vi "vacuum.vi"() -> ()   [LabVIEW 2014, in "Panels.lvlib"]
uses:
  Panels.lvlib
  CSlibraries-extern/DimLVEvent/DimIndicators/DimIndicators.lvlib
  CSCore/CSSystem/CoreLib/CoreLib.lvlib
  CSlibraries/UtilityLib/UtilityLib.valueStatus.ctl
  CSlibraries/UtilityLib/UtilityLib.lvlib
  CSCore/CSSystem/CoreLib/CoreLib.short 2 byte array.vi
  Instance           1 14Saved   vacuum .vi
  Instance           2 14Saved   vacuum .vi
  Instance           3 14Saved   vacuum .vi
  Instance           4 14Saved   vacuum .vi
  Instance           5 14Saved   vacuum .vi
  CSlibraries-extern/DimLVEvent/LVDimInterface/LVDimInterface.lvlib
  CSCore/CSSystem/CoreLib/CoreLib.string 2 byte array.vi
  CSCore/BaseProcess/BaseProcess.descriptor string definition.ctl
  CSCore/BaseProcess/BaseProcess.lvlib
  CSCore/CSSystem/CoreDefs/CoreDefs.rawDataType.ctl
  CSCore/CSSystem/CoreDefs/CoreDefs.call_type.ctl
  CSlibraries-extern/DimLVEvent/DimIndicators/DimIndicators.numericType.ctl
  CSlibraries-extern/DimLVEvent/DimIndicators/DimIndicators.numericArrayType.ctl
  CSlibraries-extern/DimLVEvent/DimIndicators/DimIndicators.anyType.ctl
panel:
  out "i ref out":refnum<vi>
  out "i ref out":refnum<vi>
  out "BOB1TP":bool
  out "BOB1TPen":bool
  in  "BOB2TISout_MonData":T1
  in  "BOB2TISin_MonData":T1
  out "BOB2TIS":bool
  in  "FVCPIR_MonData":T1={"data"=inf, "no link"=FALSE, "quality"=1, "timeStamp"=3265900746.554}
  out "FVCPIR":dbl=inf format="%.2e"
  out "LHeLevel":dbl=inf format="%.4f"
  out "LN2Level":dbl=inf format="%.4f"
  in  "LN2Level_MonData":T1={"data"=inf, "no link"=FALSE, "quality"=1, "timeStamp"=3265900746.538}
  in  "LHeLevel_MonData":T1={"data"=inf, "no link"=FALSE, "quality"=1, "timeStamp"=3265900746.554}
  in  "call cluster in":T2={"Object"="", "Selector"="", "CallType"=enum."synchronous", "Async Object"="", "Async Selector"="", "Data Descriptor"="", "Data"=[], "Error #"=0, "Expire"=0}
  in  "ReasonForLocking_SetData":T5
  in  "call cluster in":T2={"Object"="", "Selector"="", "CallType"=enum."synchronous", "Async Object"="", "Async Selector"="", "Data Descriptor"="", "Data"=[], "Error #"=0, "Expire"=0}
  in  "Reason for locking":string
  in  "BOB6_MCP_SetData":T6={"data"=[0.0, 0.0, 0.0, 0.0], "no link"=FALSE, "quality"=1, "timeStamp"=3270208307.575}
  in  "BOB6_Pho_SetData":T6={"data"=[0.0, 0.0, 0.0, 0.0], "no link"=FALSE, "quality"=1, "timeStamp"=3270208307.575}
  in  "BOB5_MCP_SetData":T6={"data"=[0.0, 0.0, 0.0, 0.0], "no link"=FALSE, "quality"=1, "timeStamp"=3270208307.575}
  in  "BOB5_Pho_SetData":T6={"data"=[0.0, 0.0, 0.0, 0.0], "no link"=FALSE, "quality"=1, "timeStamp"=3270208307.575}
  in  "BOB3_MCP_SetData":T6={"data"=[0.0, 0.0, 0.0, 0.0], "no link"=FALSE, "quality"=1, "timeStamp"=3270208307.575}
  in  "BOB3_Pho_SetData":T6={"data"=[0.0, 0.0, 0.0, 0.0], "no link"=FALSE, "quality"=1, "timeStamp"=3270208307.591}
  in  "N4VAC_MonData":T1
  in  "CB5SAFE_MonData":T1
  in  "FVAPIR_MonData":T1={"data"=inf, "no link"=FALSE, "quality"=1, "timeStamp"=3265900746.538}
  in  "FVBPIR_MonData":T1={"data"=inf, "no link"=FALSE, "quality"=1, "timeStamp"=3265900746.554}
  in  "BOB6_Pho_MonData":T1={"data"=inf, "no link"=FALSE, "quality"=1, "timeStamp"=3265900746.538}
  in  "BOB5PIR_MonData":T1={"data"=inf, "no link"=FALSE, "quality"=1, "timeStamp"=3265900746.538}
  in  "PT1PEN_MonData":T1={"data"=inf, "no link"=FALSE, "quality"=1, "timeStamp"=3265900746.538}
  in  "PT1PIR_MonData":T1={"data"=inf, "no link"=FALSE, "quality"=1, "timeStamp"=3265900746.522}
  in  "BOB6_MCP_MonData":T1={"data"=inf, "no link"=FALSE, "quality"=1, "timeStamp"=3265900746.554}
  in  "PT2PIR_MonData":T1={"data"=inf, "no link"=FALSE, "quality"=1, "timeStamp"=3265900746.569}
  in  "PT2PEN_MonData":T1={"data"=inf, "no link"=FALSE, "quality"=1, "timeStamp"=3265900746.554}
  in  "BOB1PEN_MonData":T1={"data"=inf, "no link"=FALSE, "quality"=1, "timeStamp"=3265900746.538}
  in  "BOB1PIR_MonData":T1={"data"=inf, "no link"=FALSE, "quality"=1, "timeStamp"=3265900746.569}
  in  "BOB2PEN_MonData":T1={"data"=inf, "no link"=FALSE, "quality"=1, "timeStamp"=3265900746.554}
  in  "BOB2PIR_MonData":T1={"data"=inf, "no link"=FALSE, "quality"=1, "timeStamp"=3265900746.538}
  in  "BOB3PEN_MonData":T1={"data"=inf, "no link"=FALSE, "quality"=1, "timeStamp"=3265900746.569}
  in  "BOB5PEN_MonData":T1={"data"=inf, "no link"=FALSE, "quality"=1, "timeStamp"=3265900746.569}
  in  "BOB5_Pho_MonData":T1={"data"=inf, "no link"=FALSE, "quality"=1, "timeStamp"=3265900746.538}
  in  "BOB5_MCP_MonData":T1={"data"=inf, "no link"=FALSE, "quality"=1, "timeStamp"=3265900746.585}
  in  "BOB4PIR_MonData":T1={"data"=inf, "no link"=FALSE, "quality"=1, "timeStamp"=3265900746.538}
  in  "BOB4PEN_MonData":T1={"data"=inf, "no link"=FALSE, "quality"=1, "timeStamp"=3265900746.554}
  in  "CB3PEN_MonData":T1={"data"=inf, "no link"=FALSE, "quality"=1, "timeStamp"=3265900746.569}
  in  "CB2PEN_MonData":T1={"data"=inf, "no link"=FALSE, "quality"=1, "timeStamp"=3265900746.522}
  in  "CB1PEN_MonData":T1={"data"=inf, "no link"=FALSE, "quality"=1, "timeStamp"=3265900746.538}
  in  "BOB3_Pho_MonData":T1={"data"=inf, "no link"=FALSE, "quality"=1, "timeStamp"=3265900746.6}
  in  "BOB3_MCP_MonData":T1={"data"=inf, "no link"=FALSE, "quality"=1, "timeStamp"=3265900746.585}
  in  "BOB3PIR_MonData":T1={"data"=inf, "no link"=FALSE, "quality"=1, "timeStamp"=3265900746.569}
  out "FVAPIR":dbl=inf format="%.2e"
  out "FVBPIR":dbl=inf format="%.2e"
  out "BOB6_Pho":dbl=inf format="%.3f"
  out "BOB6_MCP":dbl=inf format="%.3f"
  out "PT1PIR":dbl=inf format="%.2e"
  out "PT1PEN":dbl=inf format="%.2e"
  out "PT2PIR":dbl=inf format="%.2e"
  out "PT2PEN":dbl=inf format="%.2e"
  out "BOB5_Pho":dbl=inf format="%.3f"
  out "BOB5_MCP":dbl=inf format="%.3f"
  out "BOB5PIR":dbl=inf format="%.2e"
  out "BOB5PEN":dbl=inf format="%.2e"
  out "BOB4PIR":dbl=inf format="%.2e"
  out "BOB4PEN":dbl=inf format="%.2e"
  out "CB3PEN":dbl=inf format="%.2e"
  out "CB2PEN":dbl=inf format="%.2e"
  out "CB1PEN":dbl=inf format="%.2e"
  out "BOB3_Pho":dbl=inf format="%.3f"
  out "BOB3_MCP":dbl=inf format="%.3f"
  out "BOB3PIR":dbl=inf format="%.2e"
  out "BOB3PEN":dbl=inf format="%.2e"
  out "BOB2PIR":dbl=inf format="%.2e"
  out "BOB2PEN":dbl=inf format="%.2e"
  out "BOB1PIR":dbl=inf format="%.2e"
  out "BOB1PEN":dbl=inf format="%.2e"
  in  "BOB1FVAout_MonData":T1
  in  "BOB1FVBout_MonData":T1
  in  "BOB1GVPout_MonData":T1
  in  "BOB1GVSout_MonData":T1
  in  "BOB1BETAout_MonData":T1
  in  "BOB1TPout_MonData":T1
  in  "BOB2FCout_MonData":T1
  in  "BOB2FVAout_MonData":T1
  in  "BOB1FCout_MonData":T1
  in  "BOB2FVBout_MonData":T1
  in  "BOB2GVPout_MonData":T1
  in  "BOB2GVSout_MonData":T1
  in  "BOB2TPout_MonData":T1
  in  "TSTGVSout_MonData":T1
  in  "TSTTPout_MonData":T1
  in  "TSTFVAout_MonData":T1
  in  "TSTFVBout_MonData":T1
  in  "BOB3GVSout_MonData":T1
  in  "BOB3GVPout_MonData":T1
  in  "BOB3TPout_MonData":T1
  in  "BOB3FCout_MonData":T1
  in  "BOB3MCPout_MonData":T1
  in  "BOB3FVAout_MonData":T1
  in  "BOB3FVBout_MonData":T1
  in  "CBFVAout_MonData":T1
  in  "CBFVBout_MonData":T1
  in  "CBFVCout_MonData":T1
  in  "CB1TPout_MonData":T1
  in  "CB2TPout_MonData":T1
  in  "CB3TPout_MonData":T1
  in  "CB4TPout_MonData":T1
  in  "CB5GVSout_MonData":T1
  in  "BOB4GVSout_MonData":T1
  in  "BOB4GVPout_MonData":T1
  in  "BOB4TPout_MonData":T1
  in  "BOB4BETAout_MonData":T1
  in  "BOB4FVAout_MonData":T1
  in  "BOB4FVBout_MonData":T1
  in  "BOB5GVSout_MonData":T1
  in  "BOB5GVPout_MonData":T1
  in  "BOB5TPout_MonData":T1
  in  "BOB5FCout_MonData":T1
  in  "BOB5MCPout_MonData":T1
  in  "BOB5FVAout_MonData":T1
  in  "BOB5FVBout_MonData":T1
  in  "PT1GVPout_MonData":T1
  in  "PT1TPout_MonData":T1
  in  "PT1FVAout_MonData":T1
  in  "PT1FVBout_MonData":T1
  in  "PT2GVPout_MonData":T1
  in  "PT2TPout_MonData":T1
  in  "PT2FVAout_MonData":T1
  in  "PT2FVBout_MonData":T1
  in  "BOB2lock_SetData":T1
  in  "BOB3lock_SetData":T1
  in  "BOB4lock_SetData":T1
  in  "BOB5lock_SetData":T1
  in  "TSTlock_SetData":T1
  in  "CBlock_SetData":T1
  in  "PTlock_SetData":T1
  in  "BOB1lock_SetData":T1
  in  "PT2FVBin_MonData":T1
  in  "PT2FVAin_MonData":T1
  in  "PT2TPin_MonData":T1
  in  "PT2GVPin_MonData":T1
  in  "PT1FVBin_MonData":T1
  in  "PT1FVAin_MonData":T1
  in  "PT1TPin_MonData":T1
  in  "PT1GVPin_MonData":T1
  in  "BOB5FVBin_MonData":T1
  in  "BOB5FVAin_MonData":T1
  in  "BOB5MCPin_MonData":T1
  in  "BOB5FCin_MonData":T1
  in  "BOB5TPin_MonData":T1
  in  "BOB5GVPin_MonData":T1
  in  "BOB5GVSin_MonData":T1
  in  "BOB4FVBin_MonData":T1
  in  "BOB4FVAin_MonData":T1
  in  "BOB4BETAin_MonData":T1
  in  "BOB4TPin_MonData":T1
  in  "BOB4GVPin_MonData":T1
  in  "BOB4GVSin_MonData":T1
  in  "CB5GVSin_MonData":T1
  in  "CB4TPin_MonData":T1
  in  "CB3TPin_MonData":T1
  in  "CB2TPin_MonData":T1
  in  "CB1TPin_MonData":T1
  in  "CBFVCin_MonData":T1
  in  "CBFVBin_MonData":T1
  in  "CBFVAin_MonData":T1
  in  "BOB3FVBin_MonData":T1
  in  "BOB3FVAin_MonData":T1
  in  "BOB3MCPin_MonData":T1
  in  "BOB3FCin_MonData":T1
  in  "BOB3TPin_MonData":T1
  in  "BOB3GVPin_MonData":T1
  in  "BOB3GVSin_MonData":T1
  in  "TSTFVBin_MonData":T1
  in  "TSTFVAin_MonData":T1
  in  "TSTTPin_MonData":T1
  in  "TSTGVSin_MonData":T1
  in  "BOB2TPin_MonData":T1
  out "TSTlock":bool
  out "BOB3lock":bool
  out "BOB1BETA":bool
  out "BOB1FC":bool
  out "BOB6FC":bool
  out "BOB6MCP":bool=TRUE
  out "BOB3MCP":bool
  out "BOB3FC":bool
  out "BOB2FC":bool
  out "BOB1lock":bool
  out "BOB2lock":bool
  out "BOB5MCP":bool
  out "BOB5FC":bool
  out "BOB4BETA":bool
  out "CBlock":bool
  out "PTlock":bool
  out "BOB5lock":bool
  out "BOB4lock":bool
  out "BOB1GVS":bool
  out "TSTGVS":bool
  out "BOB2GVS":bool
  out "BOB3GVS":bool
  out "BOB4GVS":bool
  out "BOB5GVS":bool
  out "BOB1GVP":bool
  out "BOB2GVP":bool
  out "BOB3GVP":bool
  out "CB5GVS":bool
  out "BOB4GVP":bool
  out "BOB5GVP":bool
  out "PT1GVP":bool
  out "PT2GVP":bool
  out "BOB1FVA":bool
  out "BOB1FVB":bool
  out "BOB2FVA":bool
  out "BOB2FVB":bool
  out "TSTFVA":bool
  out "TSTFVB":bool
  out "BOB3FVA":bool
  out "BOB3FVB":bool
  out "CBFVA":bool
  out "CBFVC":bool
  out "CBFVB":bool
  out "BOB4FVA":bool
  out "BOB4FVB":bool
  out "BOB5FVA":bool
  out "BOB5FVB":bool
  out "PT1FVA":bool
  out "PT1FVB":bool
  out "PT2FVA":bool
  out "PT2FVB":bool
  out "CB1TP":bool
  out "BOB3TP":bool
  out "TSTTP":bool
  out "CB2TP":bool
  out "BOB2TP":bool
  out "CB5SAFE":bool=TRUE
  out "N4VAC":bool=TRUE
  out "BOB5TP":bool
  out "PT2TP":bool
  out "BOB4TP":bool
  out "PT1TP":bool
  out "CB4TP":bool
  out "CB3TP":bool
  in  "BOB2GVSin_MonData":T1
  in  "BOB2GVPin_MonData":T1
  out "i ref out":refnum<vi>
  in  "BOB1FCin_MonData":T1
  in  "BOB2FVAin_MonData":T1
  in  "BOB2FCin_MonData":T1
  in  "BOB1TPin_MonData":T1
  in  "BOB1BETAin_MonData":T1
  in  "BOB1GVSin_MonData":T1
  in  "BOB1GVPin_MonData":T1
  in  "BOB1FVBin_MonData":T1
  in  "BOB1FVAin_MonData":T1
  in  "BOB2FVBin_MonData":T1
  out "PT2FVBen":bool
  out "PT2FVAen":bool
  out "PT1FVBen":bool
  out "PT1FVAen":bool
  out "BOB5FVBen":bool
  out "BOB5FVAen":bool
  out "BOB4FVBen":bool
  out "BOB4FVAen":bool
  out "BOB3FVBen":bool
  out "BOB3FVAen":bool
  out "TSTFVBen":bool
  out "BOB2FVBen":bool
  out "TSTFVAen":bool
  out "BOB2FVAen":bool
  out "BOB1FVBen":bool
  out "BOB1FVAen":bool
  out "CBFVCen":bool
  out "CBFVBen":bool
  out "CBFVAen":bool
  out "PT2GVPen":bool
  out "PT1GVPen":bool
  out "BOB5GVPen":bool
  out "BOB4GVPen":bool
  out "BOB3GVPen":bool
  out "BOB2GVPen":bool
  out "BOB1GVPen":bool
  out "BOB5GVSen":bool
  out "BOB4GVSen":bool
  out "BOB3GVSen":bool
  out "BOB2GVSen":bool
  out "BOB1GVSen":bool
  out "TSTGVSen":bool
  out "BOB2TPen":bool
  out "TSTTPen":bool
  out "BOB3TPen":bool
  out "BOB4TPen":bool
  out "BOB5TPen":bool
  out "PT1TPen":bool
  out "PT2TPen":bool
  out "CB1TPen":bool
  out "CB5GVSen":bool
  # "voltage"
  # "V"
  # "voltage"
  # "V"
  # "N4VAC"
  # "CB5SAFE"
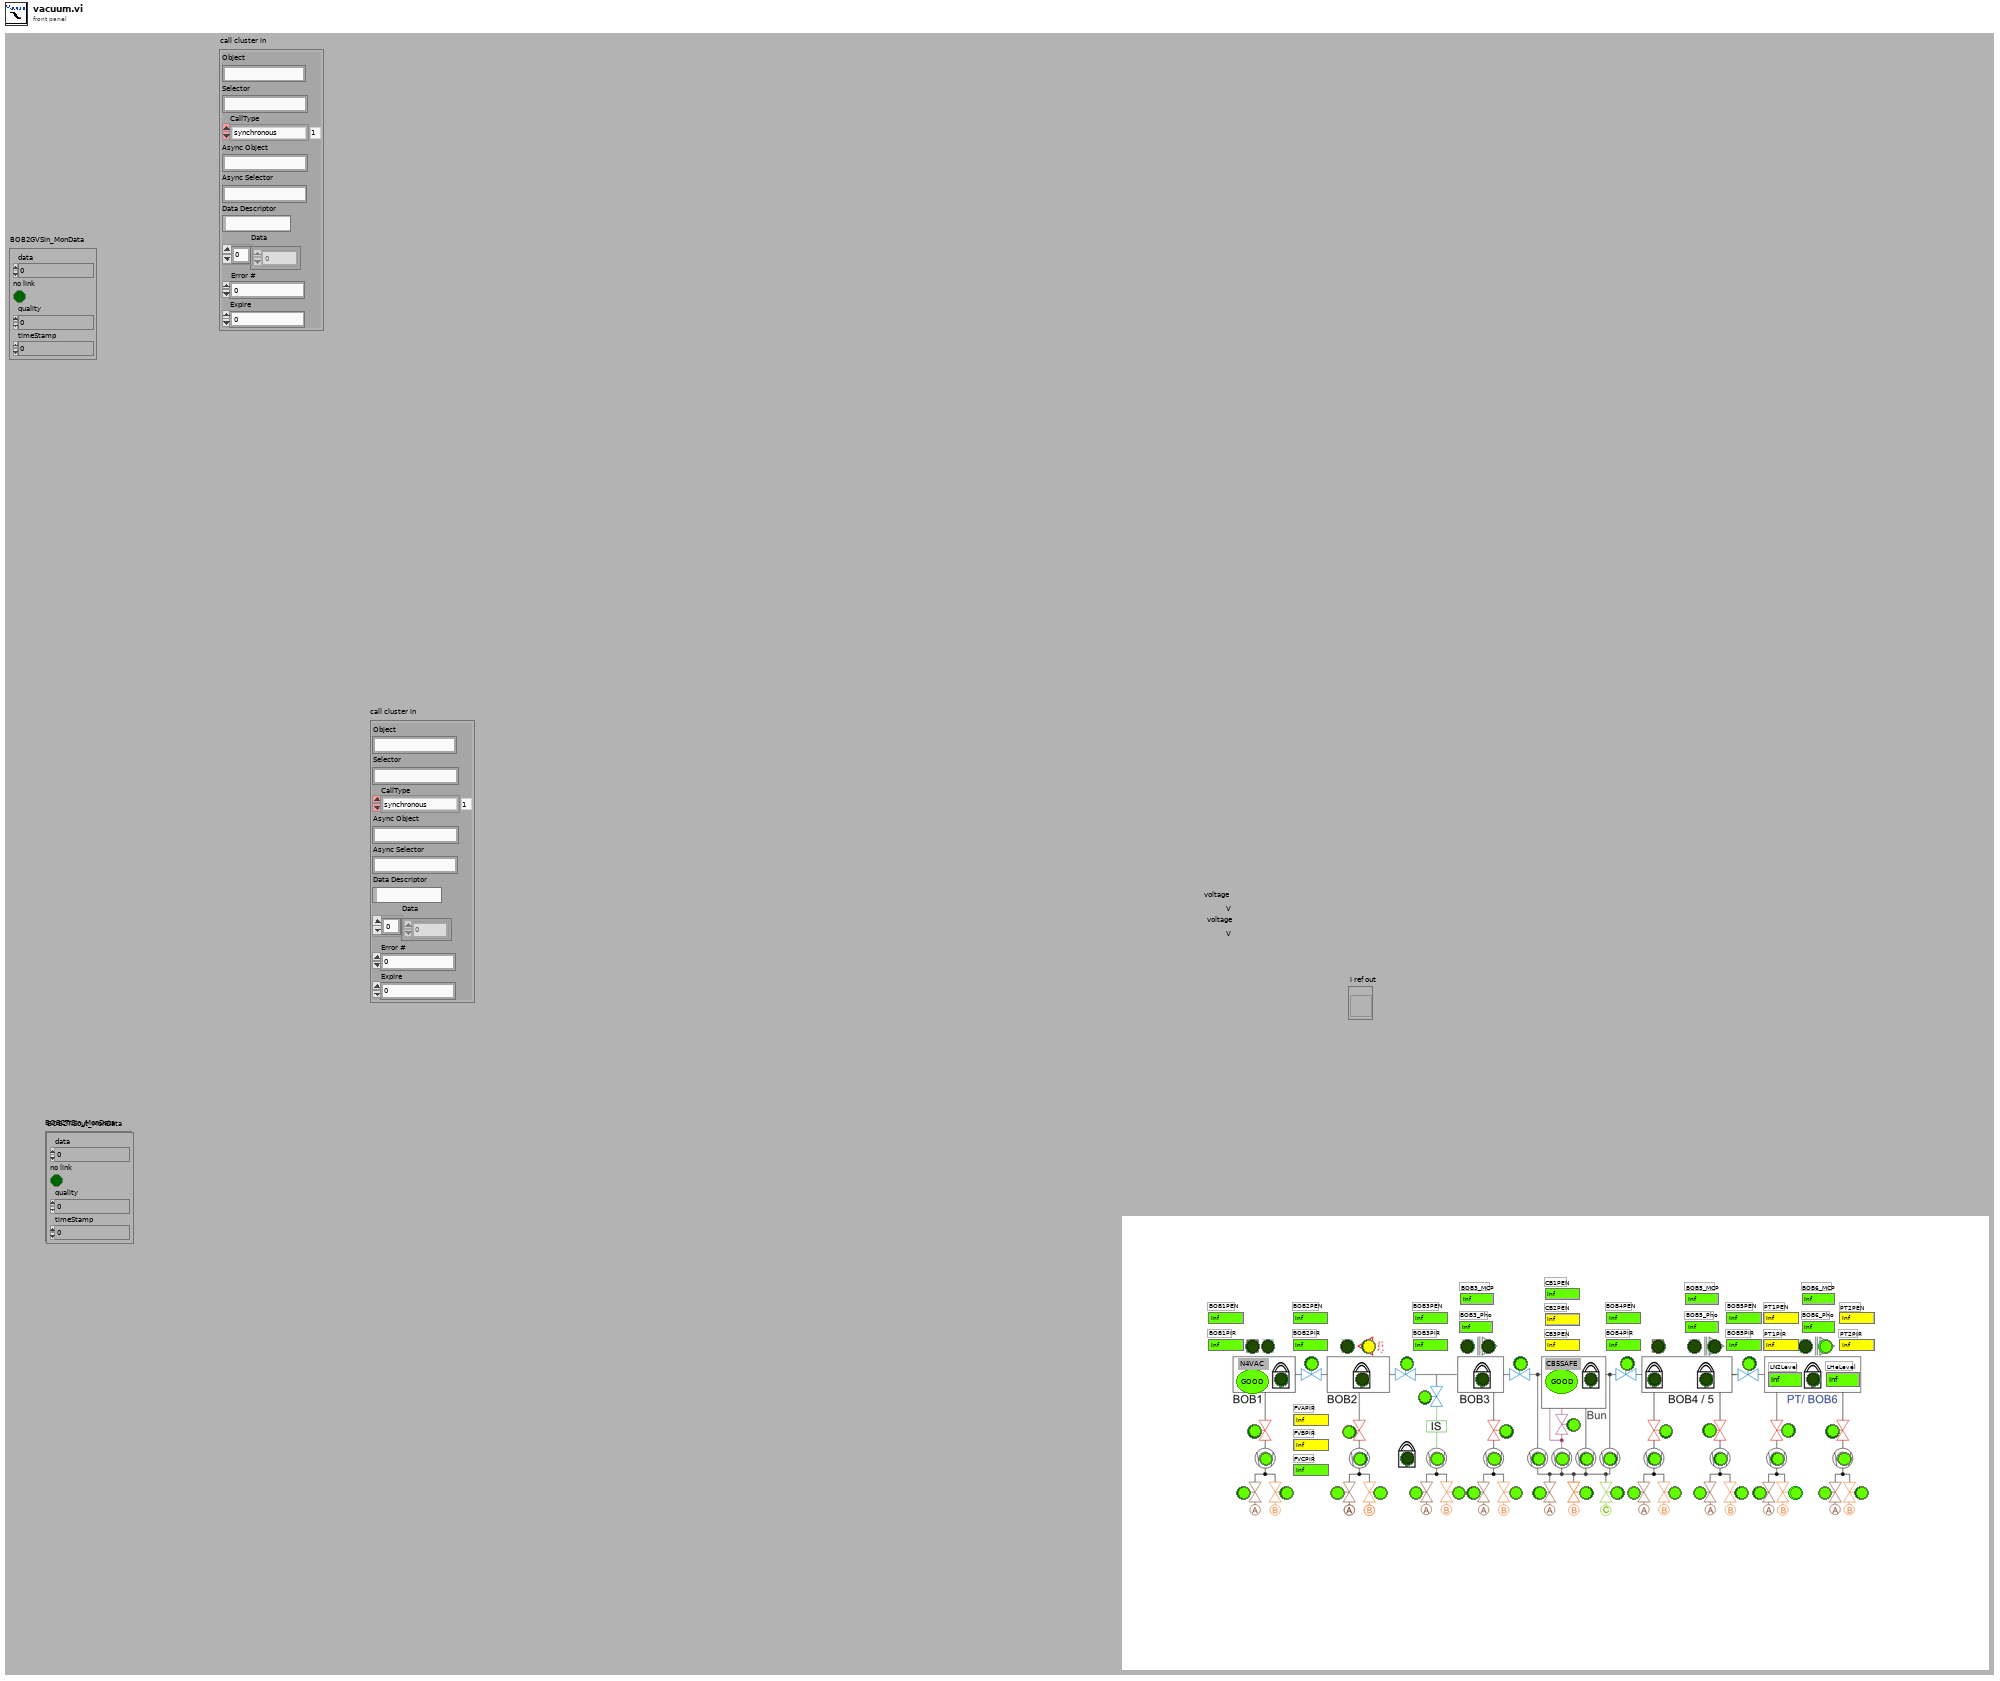
[diagram p1: front panel]
types:
  T1 = typedef "DimIndicators.lvlib/DimIndicators.numericType.ctl" = cluster{"data":dbl, "no link":bool, "quality":i32, "timeStamp":dbl}
  T2 = typedef "CoreDefs.call_type.ctl" = cluster{"Object":string, "Selector":string, "CallType":enum16{"simple", "synchronous", "asynchronous"}, "Async Object":string, "Async Selector":string, "Data Descriptor":T3, "Data":T4, "Error #":i32, "Expire":u32}
  T3 = typedef "BaseProcess.lvlib/BaseProcess.descriptor string definition.ctl" = string
  T4 = typedef "CoreDefs.rawDataType.ctl" = i8[]
  T5 = typedef "DimIndicators.lvlib/DimIndicators.anyType.ctl" = cluster{"data":string, "no link":bool, "quality":i32, "timeStamp":dbl}
  T6 = typedef "DimIndicators.lvlib/DimIndicators.numericArrayType.ctl" = cluster{"data":dbl[], "no link":bool, "quality":i32, "timeStamp":dbl}
  T7 = typedef "UtilityLib.lvlib/UtilityLib.valueStatus.ctl" = enum16{"no info available", "stand by/off", "on", "warning", "alarm/malfunction", "not implemented", "user action required", "important information", "system default", "control default", "indicator default", "button default"}
  T8 = cluster{"data":i16, "no link":bool, "quality":i32, "timeStamp":dbl}
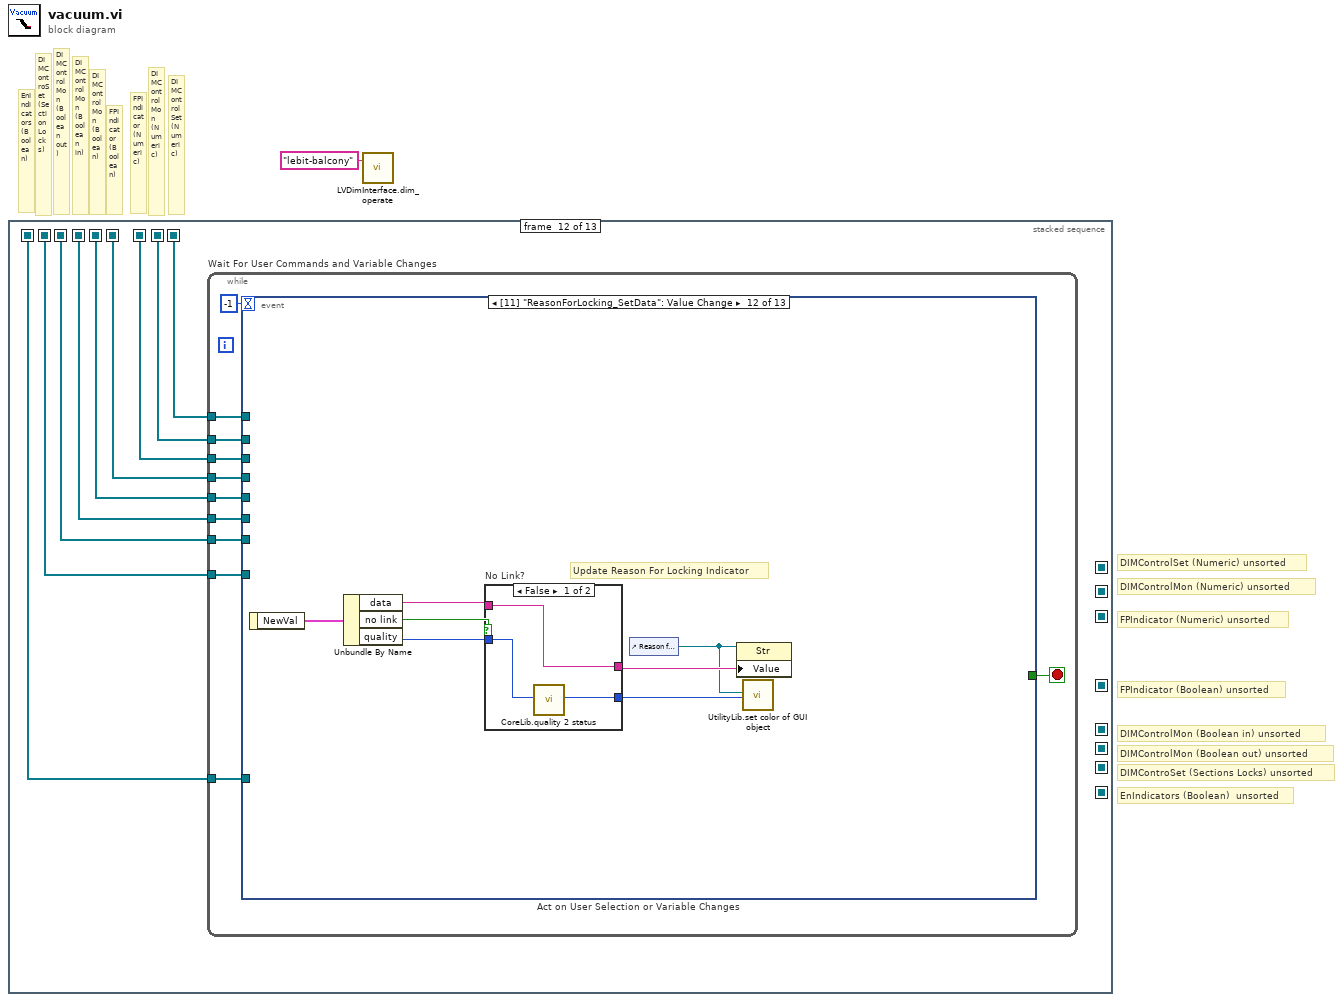
[diagram p0: block diagram]
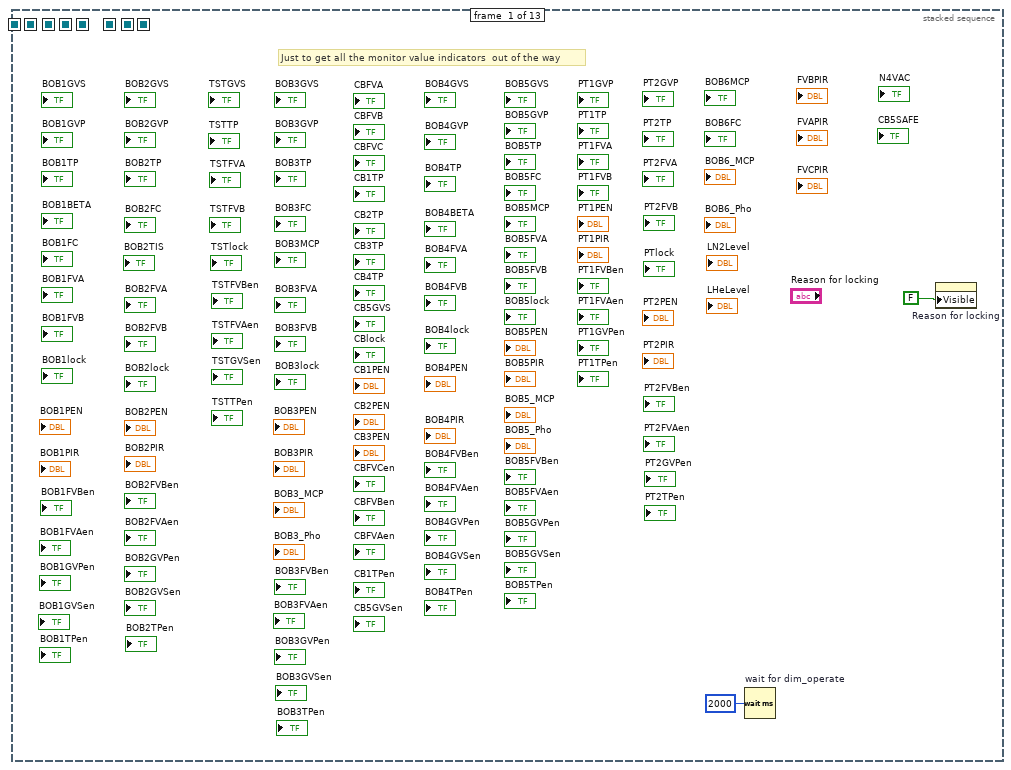
[diagram p2: hidden frame]
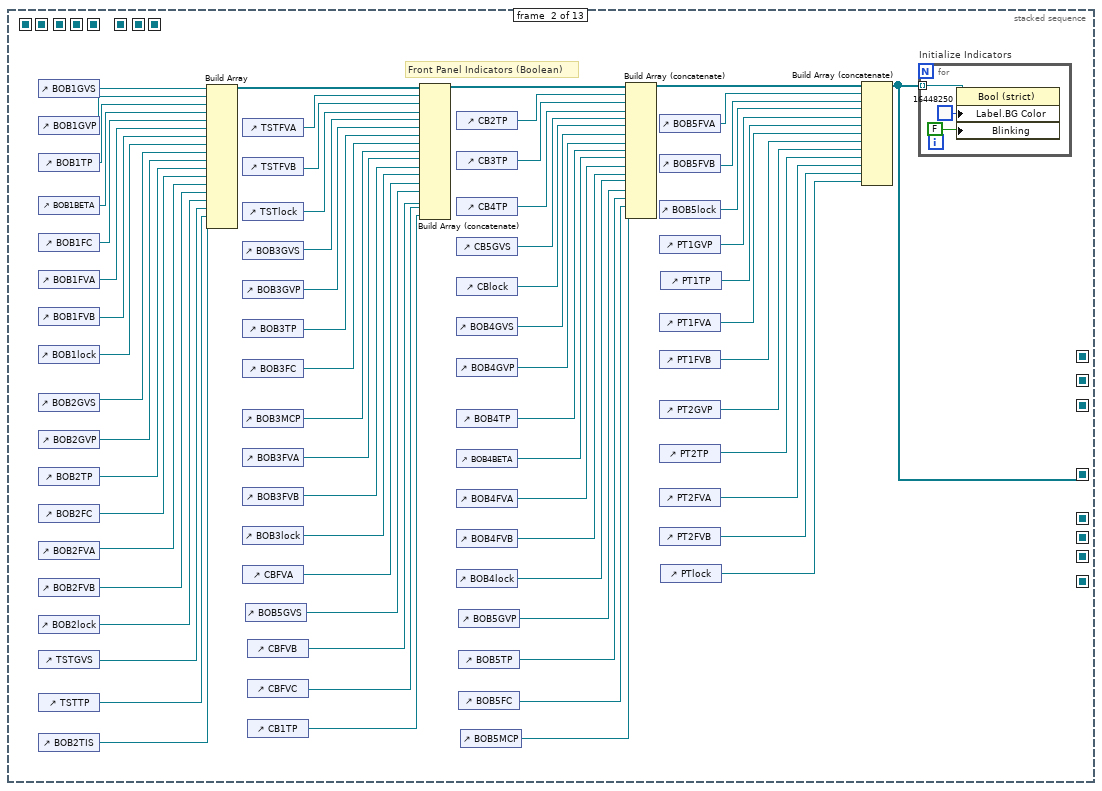
[diagram p3: hidden frame]
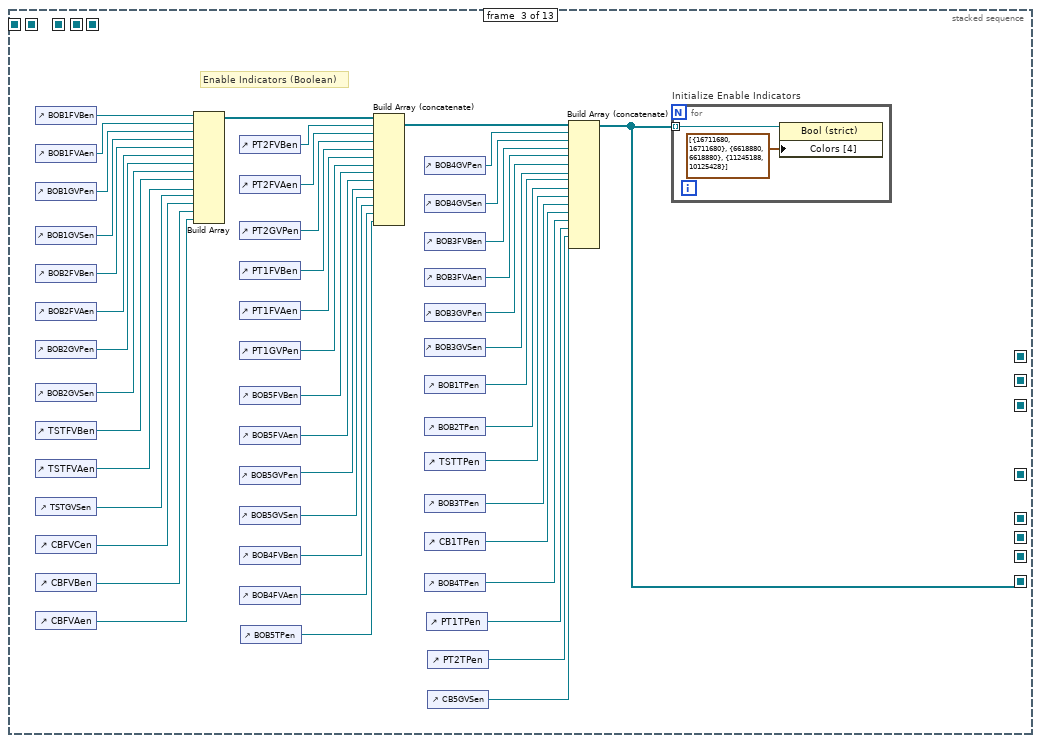
[diagram p4: hidden frame]
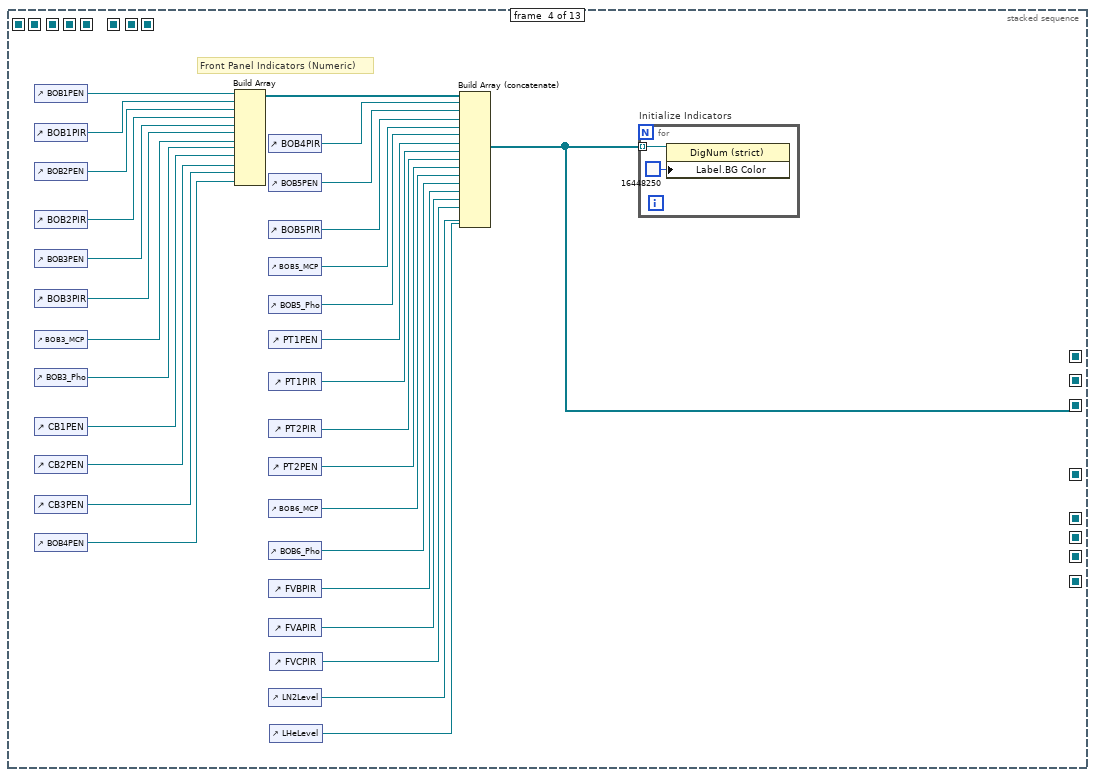
[diagram p5: hidden frame]
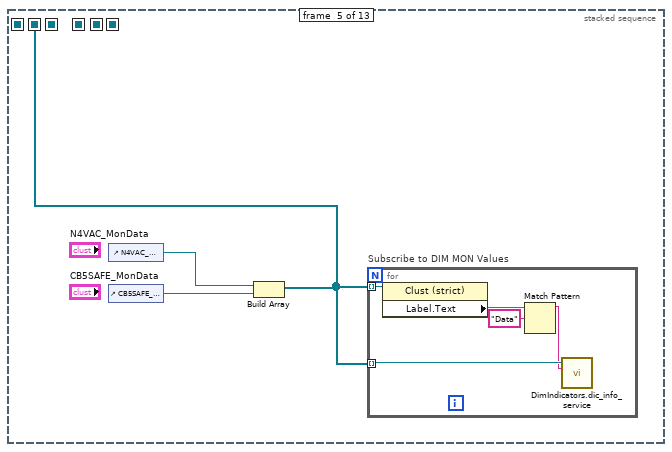
[diagram p6: hidden frame]
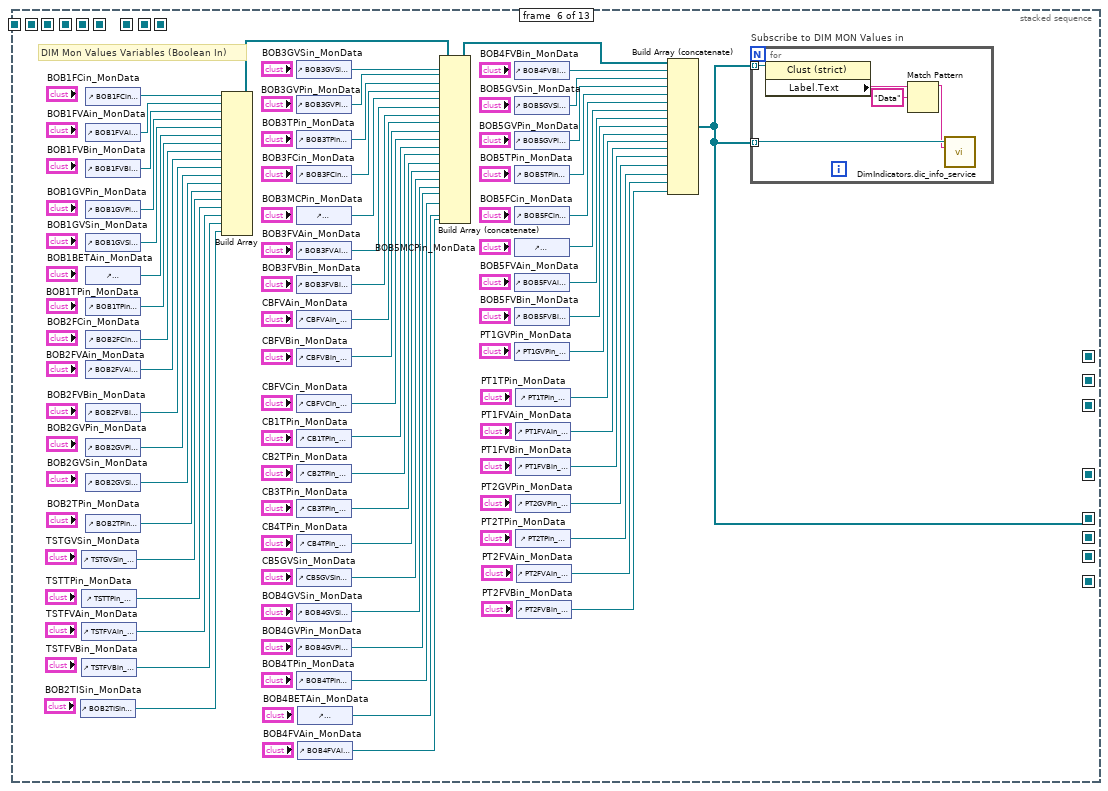
[diagram p7: hidden frame]
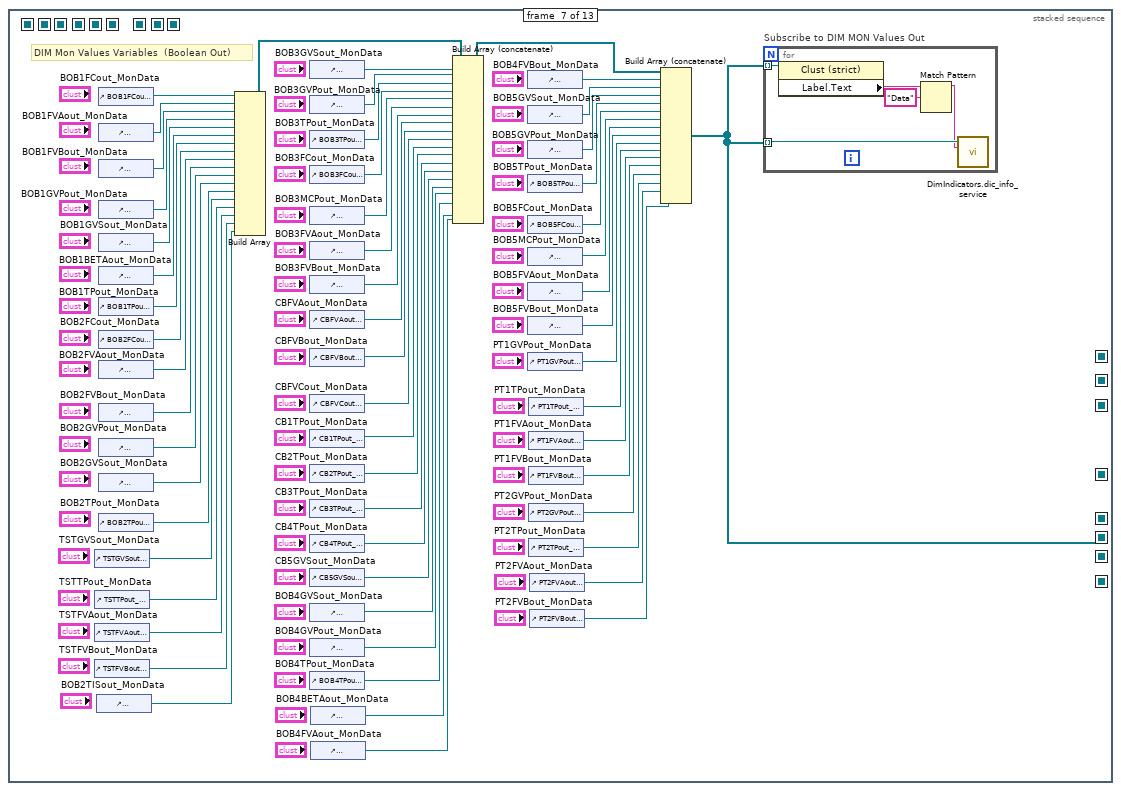
[diagram p8: hidden frame]
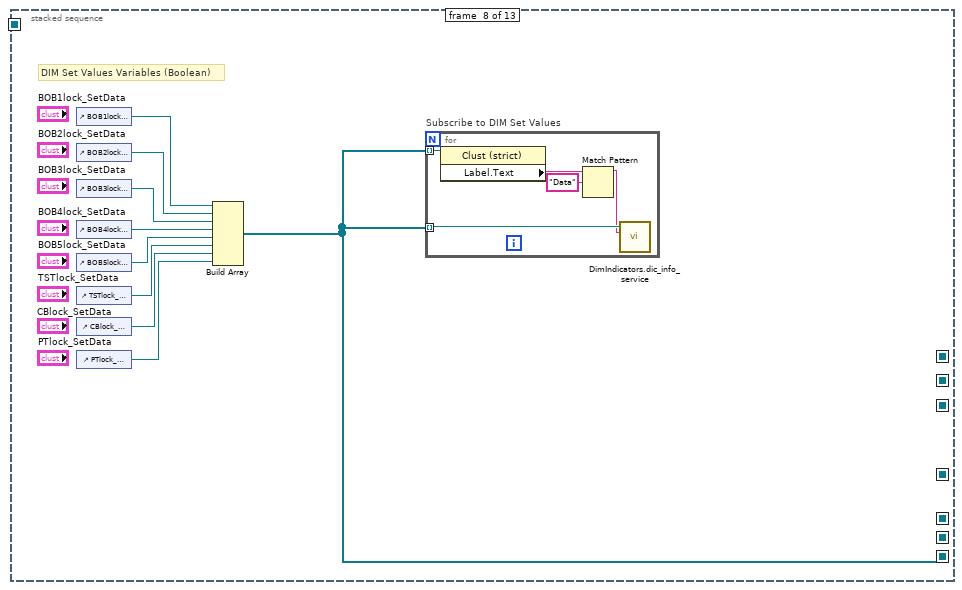
[diagram p9: hidden frame]
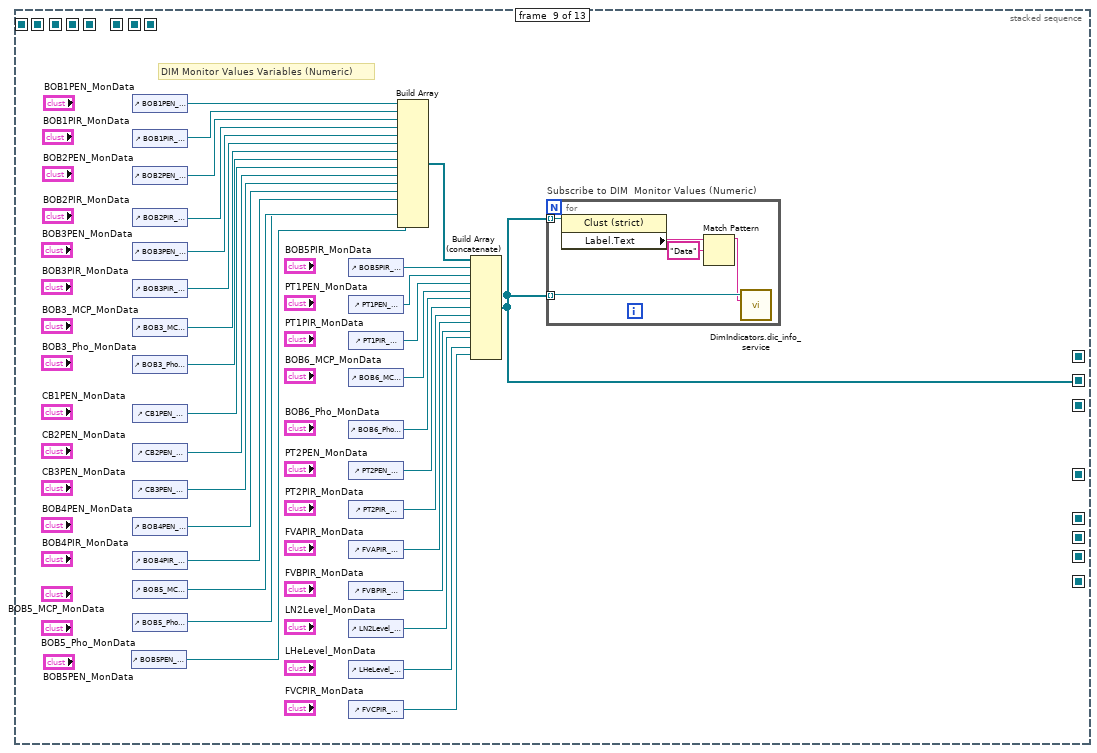
[diagram p10: hidden frame]
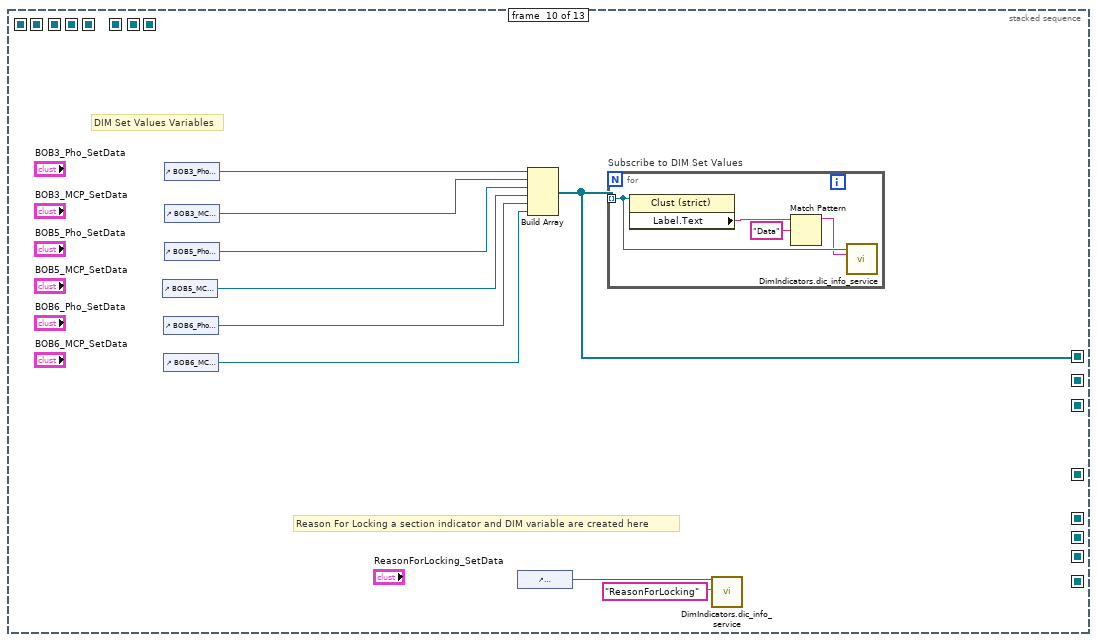
[diagram p11: hidden frame]
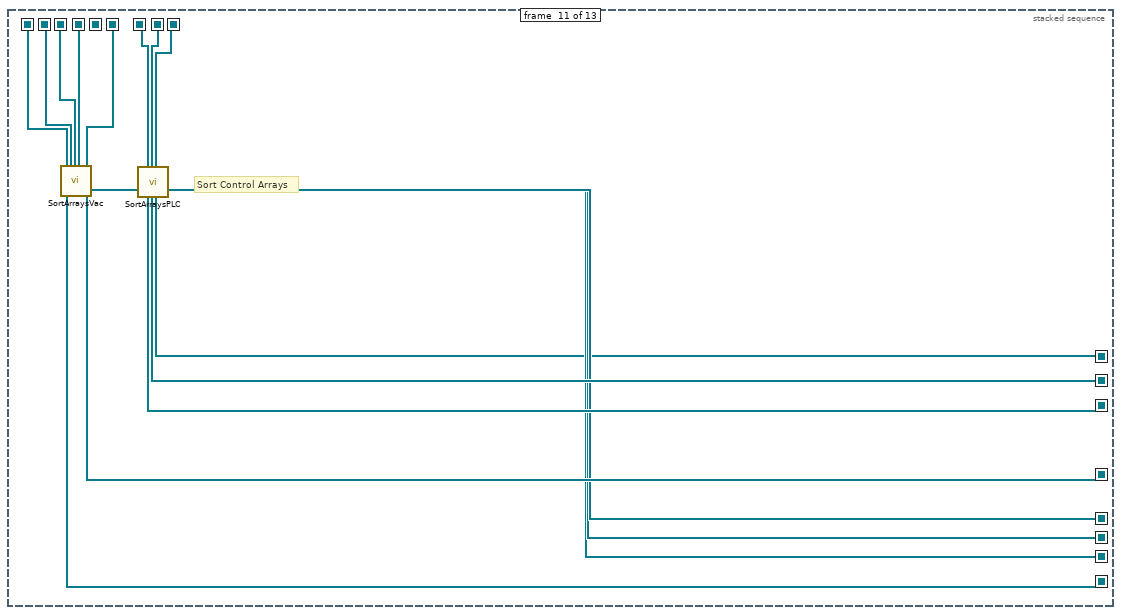
[diagram p12: hidden frame]
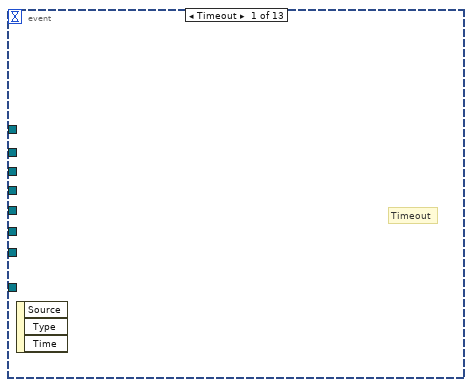
[diagram p13: hidden frame]
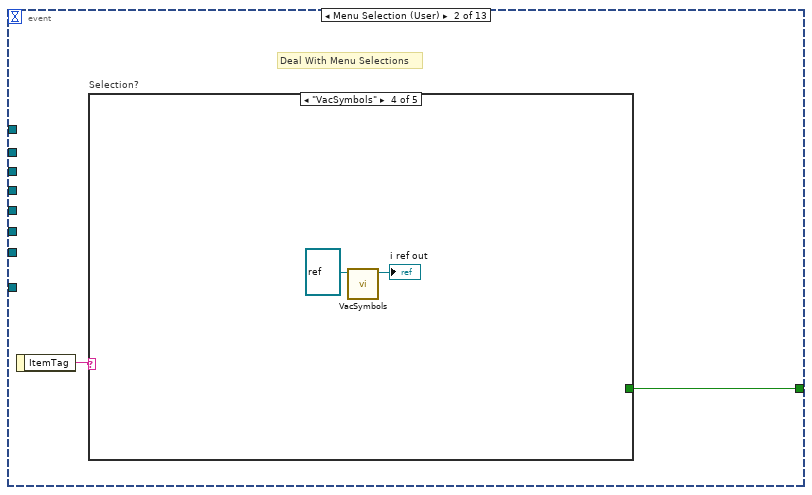
[diagram p14: hidden frame]
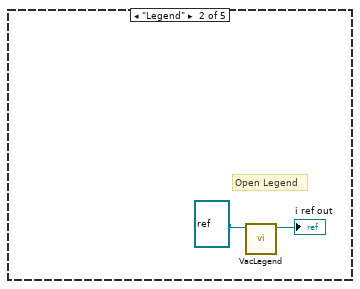
[diagram p16: hidden frame]
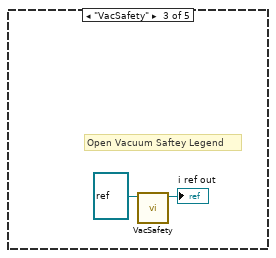
[diagram p17: hidden frame]
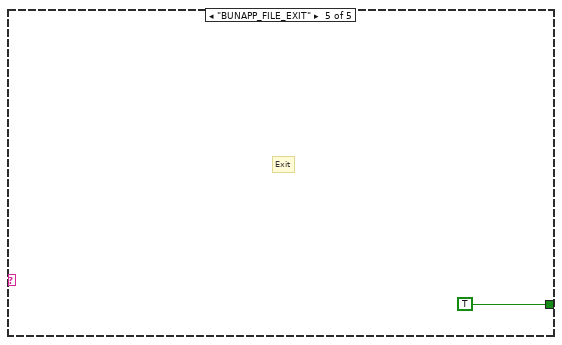
[diagram p18: hidden frame]
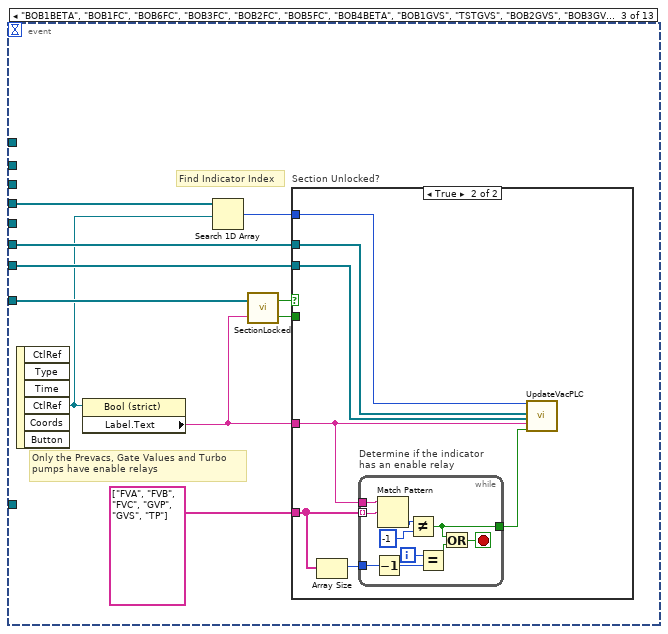
[diagram p19: hidden frame]
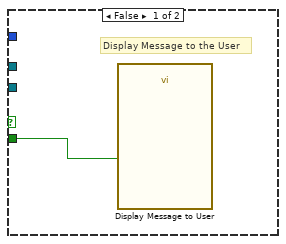
[diagram p20: hidden frame]
diagram:
  # "EnIndicators (Boolean)"
  # "EnIndicators (Boolean)  unsorted"
  # "DIMControlSet (Numeric)"
  # "DIMControlSet (Numeric) unsorted"
  # "DIMControlMon (Boolean)"
  # "DIMControlMon (Numeric) unsorted"
  # "DIMControlMon (Boolean out) unsorted"
  # "FPIndicator (Numeric) unsorted"
  # "DIMControSet (Sections Locks) unsorted"
  # "DIMControlMon (Boolean in) unsorted"
  # "FPIndicator (Boolean) unsorted"
  # "DIMControlMon (Numeric)"
  # "DIMControlMon (Boolean out)"
  # "FPIndicator (Numeric)"
  # "DIMControSet (Section Locks)"
  # "DIMControlMon (Boolean in)"
  # "FPIndicator (Boolean)"
  n1 = stacked-sequence {
    seq-local: [_ w6 _ _ _ _ _ _ _ _ _ _ _] -> [_ _ _ _ _ _ _ _ _ _ w361 _ _]
    seq-local: [_ _ _ _ _ w161 _ _ _ _ _ _ _] -> [_ _ _ _ _ _ _ _ _ _ w355 _ _]
    seq-local: [_ _ _ _ _ _ _ w284 _ _ _ _ _] -> [_ _ _ _ _ _ _ _ _ _ w353 _ _]
    seq-local: [_ _ _ w148 _ _ _ _ _ _ _ _ _] -> [_ _ _ _ _ _ _ _ _ _ w359 _ _]
    seq-local: [_ _ _ _ _ _ w223 _ _ _ _ _ _] -> [_ _ _ _ _ _ _ _ _ _ w354 _ _]
    seq-local: [_ _ _ _ _ _ _ _ w301 _ _ _ _] -> [_ _ _ _ _ _ _ _ _ _ w358 _ _]
    seq-local: [_ _ _ _ _ _ _ _ _ _ w356 _ _] -> [_ _ _ _ _ _ _ _ _ _ _ w369 w825]
    seq-local: [_ _ _ _ _ _ _ _ _ _ w352 _ _] -> [_ _ _ _ _ _ _ _ _ _ _ w366 w822]
    seq-local: [_ _ _ _ _ _ _ _ _ _ w350 _ _] -> [_ _ _ _ _ _ _ _ _ _ _ w367 w823]
    seq-local: [_ _ _ _ _ _ _ _ _ _ w351 _ _] -> [_ _ _ _ _ _ _ _ _ _ _ w368 w824]
    seq-local: [_ _ _ _ _ _ _ _ _ _ w357 _ _] -> [_ _ _ _ _ _ _ _ _ _ _ w370 _]
    seq-local: [_ _ _ _ _ _ _ _ _ _ w360 _ _] -> [_ _ _ _ _ _ _ _ _ _ _ w365 _]
    seq-local: [_ _ _ _ w152 _ _ _ _ _ _ _ _] -> [_ _ _ _ _ _ _ _ _ _ _ w364 w820]
    seq-local: [_ _ _ _ _ _ _ _ _ w335 _ _ _] -> [_ _ _ _ _ _ _ _ _ _ w349 _ _]
    seq-local: [_ _ _ _ _ _ _ _ _ _ w348 _ _] -> [_ _ _ _ _ _ _ _ _ _ _ w363 w821]
    seq-local: [_ _ w83 _ _ _ _ _ _ _ _ _ _] -> [_ _ _ _ _ _ _ _ _ _ w347 _ _]
    seq-local: [_ _ _ _ _ _ _ _ _ _ w346 _ _] -> [_ _ _ _ _ _ _ _ _ _ _ w362 _]
    frame #0 {
      # "Just to get all the monitor value indicators  out of the way"
      n2 = Wait (ms) "wait for dim_operate"(milliseconds to wait=u32 2000) -> ()  [unwired: 1 out]
      n3 = property on="Reason for locking" class="Str"("Visible"=FALSE) -> ()  [unwired: 2 in, 2 out]
    }
    frame #1 {
      # "Front Panel Indicators (Boolean)"
      # "Arrange references to all monitor-value related buttons into an array."
      n4 = control-ref of="BOB1GVS"() -> (w69:refnum<vi>)
      n5 = control-ref of="BOB1GVP"() -> (w68:refnum<vi>)
      n6 = control-ref of="BOB1TP"() -> (w67:refnum<vi>)
      n7 = control-ref of="BOB1BETA"() -> (w66:refnum<vi>)
      n8 = control-ref of="BOB1FC"() -> (w65:refnum<vi>)
      n9 = control-ref of="BOB1FVA"() -> (w64:refnum<vi>)
      n10 = control-ref of="BOB1FVB"() -> (w63:refnum<vi>)
      n11 = control-ref of="BOB1lock"() -> (w62:refnum<vi>)
      n12 = control-ref of="BOB2GVS"() -> (w61:refnum<vi>)
      n13 = control-ref of="BOB2GVP"() -> (w60:refnum<vi>)
      n14 = control-ref of="BOB2TP"() -> (w59:refnum<vi>)
      n15 = control-ref of="BOB2FC"() -> (w58:refnum<vi>)
      n16 = control-ref of="BOB2FVA"() -> (w57:refnum<vi>)
      n17 = control-ref of="BOB2FVB"() -> (w56:refnum<vi>)
      n18 = control-ref of="BOB2lock"() -> (w55:refnum<vi>)
      n19 = control-ref of="TSTGVS"() -> (w54:refnum<vi>)
      n20 = control-ref of="TSTTP"() -> (w53:refnum<vi>)
      n21 = control-ref of="BOB2TIS"() -> (w4:refnum<vi>)
      n22 = Build Array(w69, w68, w67, w66, w65, w64, w63, w62, w61, w60, w59, w58, w57, w56, w55, w54, w53, w4) -> (w52:refnum<vi>[])
      n23 = control-ref of="TSTFVA"() -> (w51:refnum<vi>)
      n24 = control-ref of="TSTFVB"() -> (w50:refnum<vi>)
      n25 = control-ref of="TSTlock"() -> (w49:refnum<vi>)
      n26 = control-ref of="BOB3GVS"() -> (w48:refnum<vi>)
      n27 = control-ref of="BOB3GVP"() -> (w47:refnum<vi>)
      n28 = control-ref of="BOB3TP"() -> (w46:refnum<vi>)
      n29 = control-ref of="BOB3FC"() -> (w45:refnum<vi>)
      n30 = control-ref of="BOB3MCP"() -> (w44:refnum<vi>)
      n31 = control-ref of="BOB3FVA"() -> (w43:refnum<vi>)
      n32 = control-ref of="BOB3FVB"() -> (w42:refnum<vi>)
      n33 = control-ref of="BOB3lock"() -> (w41:refnum<vi>)
      n34 = control-ref of="CBFVA"() -> (w40:refnum<vi>)
      n35 = control-ref of="BOB5GVS"() -> (w39:refnum<vi>)
      n36 = control-ref of="CBFVB"() -> (w38:refnum<vi>)
      n37 = control-ref of="CBFVC"() -> (w37:refnum<vi>)
      n38 = control-ref of="CB1TP"() -> (w36:refnum<vi>)
      n39 = Build Array (concatenate)(w52, w51, w50, w49, w48, w47, w46, w45, w44, w43, w42, w41, w40, w39, w38, w37, w36) -> (w35:refnum<vi>[])
      n40 = control-ref of="CB2TP"() -> (w34:refnum<vi>)
      n41 = control-ref of="CB3TP"() -> (w33:refnum<vi>)
      n42 = control-ref of="CB4TP"() -> (w32:refnum<vi>)
      n43 = control-ref of="CB5GVS"() -> (w31:refnum<vi>)
      n44 = control-ref of="CBlock"() -> (w30:refnum<vi>)
      n45 = control-ref of="BOB4GVS"() -> (w29:refnum<vi>)
      n46 = control-ref of="BOB4GVP"() -> (w28:refnum<vi>)
      n47 = control-ref of="BOB4TP"() -> (w27:refnum<vi>)
      n48 = control-ref of="BOB4BETA"() -> (w26:refnum<vi>)
      n49 = control-ref of="BOB4FVA"() -> (w25:refnum<vi>)
      n50 = control-ref of="BOB4FVB"() -> (w24:refnum<vi>)
      n51 = control-ref of="BOB4lock"() -> (w23:refnum<vi>)
      n52 = control-ref of="BOB5GVP"() -> (w22:refnum<vi>)
      n53 = control-ref of="BOB5TP"() -> (w21:refnum<vi>)
      n54 = control-ref of="BOB5FC"() -> (w20:refnum<vi>)
      n55 = control-ref of="BOB5MCP"() -> (w19:refnum<vi>)
      n56 = Build Array (concatenate)(w35, w34, w33, w32, w31, w30, w29, w28, w27, w26, w25, w24, w23, w22, w21, w20, w19) -> (w18:refnum<vi>[])
      n57 = control-ref of="BOB5FVA"() -> (w17:refnum<vi>)
      n58 = control-ref of="BOB5FVB"() -> (w16:refnum<vi>)
      n59 = control-ref of="BOB5lock"() -> (w15:refnum<vi>)
      n60 = control-ref of="PT1GVP"() -> (w14:refnum<vi>)
      n61 = control-ref of="PT1FVA"() -> (w13:refnum<vi>)
      n62 = control-ref of="PT1FVB"() -> (w12:refnum<vi>)
      n63 = control-ref of="PT2GVP"() -> (w11:refnum<vi>)
      n64 = control-ref of="PT2TP"() -> (w10:refnum<vi>)
      n65 = control-ref of="PT2FVA"() -> (w9:refnum<vi>)
      n66 = control-ref of="PT2FVB"() -> (w8:refnum<vi>)
      n67 = control-ref of="PT1TP"() -> (w5:refnum<vi>)
      n68 = control-ref of="PTlock"() -> (w7:refnum<vi>)
      n69 = Build Array (concatenate)(w18, w17, w16, w15, w14, w5, w13, w12, w11, w10, w9, w8, w7) -> (w6:refnum<vi>[])
      n70 = for "Initialize Indicators" {
        tunnel: w6 -> [w72] mode=indexing
        n71 = property class="Bool (strict)"(reference=w72, "Label.BG Color"=u32 16448250 ("Color Box"), "Blinking"=FALSE) -> ()  [unwired: 1 in, 2 out]
      }
    }
    frame #2 {
      # "Enable Indicators (Boolean)"
      n72 = control-ref of="BOB1FVBen"() -> (w117:refnum<vi>)
      n73 = control-ref of="BOB1FVAen"() -> (w116:refnum<vi>)
      n74 = control-ref of="BOB1GVPen"() -> (w115:refnum<vi>)
      n75 = control-ref of="BOB1GVSen"() -> (w114:refnum<vi>)
      n76 = control-ref of="BOB2FVBen"() -> (w113:refnum<vi>)
      n77 = control-ref of="BOB2FVAen"() -> (w112:refnum<vi>)
      n78 = control-ref of="BOB2GVPen"() -> (w111:refnum<vi>)
      n79 = control-ref of="BOB2GVSen"() -> (w110:refnum<vi>)
      n80 = control-ref of="TSTFVBen"() -> (w109:refnum<vi>)
      n81 = control-ref of="TSTFVAen"() -> (w108:refnum<vi>)
      n82 = control-ref of="TSTGVSen"() -> (w107:refnum<vi>)
      n83 = control-ref of="CBFVCen"() -> (w106:refnum<vi>)
      n84 = control-ref of="CBFVBen"() -> (w105:refnum<vi>)
      n85 = control-ref of="CBFVAen"() -> (w104:refnum<vi>)
      n86 = Build Array(w117, w116, w115, w114, w113, w112, w111, w110, w109, w108, w107, w106, w105, w104) -> (w103:refnum<vi>[])
      n87 = control-ref of="PT2FVBen"() -> (w102:refnum<vi>)
      n88 = control-ref of="PT2FVAen"() -> (w101:refnum<vi>)
      n89 = control-ref of="PT2GVPen"() -> (w100:refnum<vi>)
      n90 = control-ref of="PT1FVBen"() -> (w99:refnum<vi>)
      n91 = control-ref of="PT1FVAen"() -> (w98:refnum<vi>)
      n92 = control-ref of="PT1GVPen"() -> (w97:refnum<vi>)
      n93 = control-ref of="BOB5FVBen"() -> (w96:refnum<vi>)
      n94 = control-ref of="BOB5FVAen"() -> (w95:refnum<vi>)
      n95 = control-ref of="BOB5GVPen"() -> (w94:refnum<vi>)
      n96 = control-ref of="BOB5GVSen"() -> (w93:refnum<vi>)
      n97 = control-ref of="BOB4FVBen"() -> (w92:refnum<vi>)
      n98 = control-ref of="BOB4FVAen"() -> (w91:refnum<vi>)
      n99 = control-ref of="BOB5TPen"() -> (w76:refnum<vi>)
      n100 = Build Array (concatenate)(w103, w102, w101, w100, w99, w98, w97, w96, w95, w94, w93, w92, w91, w76) -> (w90:refnum<vi>[])
      n101 = control-ref of="BOB4GVPen"() -> (w89:refnum<vi>)
      n102 = control-ref of="BOB4GVSen"() -> (w88:refnum<vi>)
      n103 = control-ref of="BOB3FVBen"() -> (w87:refnum<vi>)
      n104 = control-ref of="BOB3FVAen"() -> (w86:refnum<vi>)
      n105 = control-ref of="BOB3GVPen"() -> (w85:refnum<vi>)
      n106 = control-ref of="BOB3GVSen"() -> (w84:refnum<vi>)
      n107 = control-ref of="BOB1TPen"() -> (w82:refnum<vi>)
      n108 = control-ref of="BOB2TPen"() -> (w81:refnum<vi>)
      n109 = control-ref of="TSTTPen"() -> (w80:refnum<vi>)
      n110 = control-ref of="BOB3TPen"() -> (w79:refnum<vi>)
      n111 = control-ref of="CB1TPen"() -> (w78:refnum<vi>)
      n112 = control-ref of="BOB4TPen"() -> (w77:refnum<vi>)
      n113 = control-ref of="PT1TPen"() -> (w75:refnum<vi>)
      n114 = control-ref of="PT2TPen"() -> (w74:refnum<vi>)
      n115 = control-ref of="CB5GVSen"() -> (w73:refnum<vi>)
      n116 = Build Array (concatenate)(w90, w89, w88, w87, w86, w85, w84, w82, w81, w80, w79, w78, w77, w75, w74, w73) -> (w83:refnum<vi>[])
      n117 = for "Initialize Enable Indicators" {
        tunnel: w83 -> [w119] mode=indexing
        n118 = property class="Bool (strict)"(reference=w119, "Colors [4]"=cluster{u32, u32}[] [{16711680, 16711680}, {6618880, 6618880}, {11245188, 10125428}]) -> ()  [unwired: 1 in, 2 out]
      }
    }
    frame #3 {
      # "Front Panel Indicators (Numeric)"
      n119 = control-ref of="BOB1PEN"() -> (w147:refnum<vi>)
      n120 = control-ref of="BOB1PIR"() -> (w146:refnum<vi>)
      n121 = control-ref of="BOB2PEN"() -> (w145:refnum<vi>)
      n122 = control-ref of="BOB2PIR"() -> (w144:refnum<vi>)
      n123 = control-ref of="BOB3PEN"() -> (w143:refnum<vi>)
      n124 = control-ref of="BOB3PIR"() -> (w142:refnum<vi>)
      n125 = control-ref of="BOB3_MCP"() -> (w141:refnum<vi>)
      n126 = control-ref of="BOB3_Pho"() -> (w140:refnum<vi>)
      n127 = control-ref of="CB1PEN"() -> (w139:refnum<vi>)
      n128 = control-ref of="CB2PEN"() -> (w138:refnum<vi>)
      n129 = control-ref of="CB3PEN"() -> (w137:refnum<vi>)
      n130 = control-ref of="BOB4PEN"() -> (w136:refnum<vi>)
      n131 = Build Array(w147, w146, w145, w144, w143, w142, w141, w140, w139, w138, w137, w136) -> (w149:refnum<vi>[])
      n132 = control-ref of="BOB4PIR"() -> (w135:refnum<vi>)
      n133 = control-ref of="BOB5PEN"() -> (w134:refnum<vi>)
      n134 = control-ref of="BOB5PIR"() -> (w133:refnum<vi>)
      n135 = control-ref of="BOB5_MCP"() -> (w132:refnum<vi>)
      n136 = control-ref of="BOB5_Pho"() -> (w131:refnum<vi>)
      n137 = control-ref of="PT1PEN"() -> (w130:refnum<vi>)
      n138 = control-ref of="PT1PIR"() -> (w129:refnum<vi>)
      n139 = control-ref of="PT2PIR"() -> (w128:refnum<vi>)
      n140 = control-ref of="PT2PEN"() -> (w123:refnum<vi>)
      n141 = control-ref of="BOB6_MCP"() -> (w124:refnum<vi>)
      n142 = control-ref of="BOB6_Pho"() -> (w125:refnum<vi>)
      n143 = control-ref of="FVBPIR"() -> (w126:refnum<vi>)
      n144 = control-ref of="FVAPIR"() -> (w127:refnum<vi>)
      n145 = control-ref of="LN2Level"() -> (w121:refnum<vi>)
      n146 = control-ref of="FVCPIR"() -> (w122:refnum<vi>)
      n147 = control-ref of="LHeLevel"() -> (w120:refnum<vi>)
      n148 = Build Array (concatenate)(w149, w135, w134, w133, w132, w131, w130, w129, w128, w123, w124, w125, w126, w127, w122, w121, w120) -> (w148:refnum<vi>[])
      n149 = for "Initialize Indicators" {
        tunnel: w148 -> [w151] mode=indexing
        n150 = property class="DigNum (strict)"(reference=w151, "Label.BG Color"=u32 16448250 ("Color Box")) -> ()  [unwired: 1 in, 2 out]
      }
    }
    frame #4 {
      n151 = control-ref of="N4VAC_MonData"() -> (w154:refnum<vi>)
      n152 = control-ref of="CB5SAFE_MonData"() -> (w153:refnum<vi>)
      n153 = Build Array(w154, w153) -> (w152:refnum<vi>[])
      n154 = for "Subscribe to DIM MON Values" {
        tunnel: w152 -> [w155] mode=indexing
        tunnel: w152 -> [w159] mode=indexing
        n155 = property class="Clust (strict)"(reference=w155) -> ("Label.Text"=w158:string)  [unwired: 1 in, 2 out]
        n156 = Match Pattern(string=w158, regular expression="Data") -> (before substring=w156:string)  [unwired: 1 in, 3 out]
        n157 = call "DimIndicators.dic_info_service.vi"("controlRef"=w159, "serviceName"=w156) -> ()  [unwired: 16 in, 2 out]
      }
    }
    frame #5 {
      # "DIM Mon Values Variables (Boolean In)"
      n158 = control-ref of="BOB2TISin_MonData"() -> (w160:refnum<vi>)
      n159 = control-ref of="TSTGVSin_MonData"() -> (w203:refnum<vi>)
      n160 = control-ref of="TSTTPin_MonData"() -> (w202:refnum<vi>)
      n161 = control-ref of="TSTFVAin_MonData"() -> (w201:refnum<vi>)
      n162 = control-ref of="TSTFVBin_MonData"() -> (w200:refnum<vi>)
      n163 = control-ref of="BOB1FCin_MonData"() -> (w216:refnum<vi>)
      n164 = control-ref of="BOB1FVAin_MonData"() -> (w215:refnum<vi>)
      n165 = control-ref of="BOB1FVBin_MonData"() -> (w214:refnum<vi>)
      n166 = control-ref of="BOB1GVPin_MonData"() -> (w213:refnum<vi>)
      n167 = control-ref of="BOB1GVSin_MonData"() -> (w212:refnum<vi>)
      n168 = control-ref of="BOB1BETAin_MonData"() -> (w211:refnum<vi>)
      n169 = control-ref of="BOB1TPin_MonData"() -> (w210:refnum<vi>)
      n170 = control-ref of="BOB2FCin_MonData"() -> (w209:refnum<vi>)
      n171 = control-ref of="BOB2FVAin_MonData"() -> (w208:refnum<vi>)
      n172 = control-ref of="BOB2FVBin_MonData"() -> (w207:refnum<vi>)
      n173 = control-ref of="BOB2GVPin_MonData"() -> (w206:refnum<vi>)
      n174 = control-ref of="BOB2GVSin_MonData"() -> (w205:refnum<vi>)
      n175 = control-ref of="BOB2TPin_MonData"() -> (w204:refnum<vi>)
      n176 = Build Array(w216, w215, w214, w213, w212, w211, w210, w209, w208, w207, w206, w205, w204, w203, w202, w201, w200, w160) -> (w198:refnum<vi>[])
      n177 = control-ref of="BOB3GVSin_MonData"() -> (w199:refnum<vi>)
      n178 = control-ref of="BOB3GVPin_MonData"() -> (w197:refnum<vi>)
      n179 = control-ref of="BOB3TPin_MonData"() -> (w196:refnum<vi>)
      n180 = control-ref of="BOB3FCin_MonData"() -> (w195:refnum<vi>)
      n181 = control-ref of="BOB3MCPin_MonData"() -> (w194:refnum<vi>)
      n182 = control-ref of="BOB3FVAin_MonData"() -> (w193:refnum<vi>)
      n183 = control-ref of="BOB3FVBin_MonData"() -> (w192:refnum<vi>)
      n184 = control-ref of="CBFVAin_MonData"() -> (w191:refnum<vi>)
      n185 = control-ref of="CBFVBin_MonData"() -> (w190:refnum<vi>)
      n186 = control-ref of="CBFVCin_MonData"() -> (w189:refnum<vi>)
      n187 = control-ref of="CB1TPin_MonData"() -> (w188:refnum<vi>)
      n188 = control-ref of="CB2TPin_MonData"() -> (w187:refnum<vi>)
      n189 = control-ref of="CB3TPin_MonData"() -> (w186:refnum<vi>)
      n190 = control-ref of="CB4TPin_MonData"() -> (w185:refnum<vi>)
      n191 = control-ref of="CB5GVSin_MonData"() -> (w184:refnum<vi>)
      n192 = control-ref of="BOB4GVSin_MonData"() -> (w183:refnum<vi>)
      n193 = control-ref of="BOB4GVPin_MonData"() -> (w182:refnum<vi>)
      n194 = control-ref of="BOB4TPin_MonData"() -> (w181:refnum<vi>)
      n195 = control-ref of="BOB4BETAin_MonData"() -> (w180:refnum<vi>)
      n196 = control-ref of="BOB4FVAin_MonData"() -> (w179:refnum<vi>)
      n197 = Build Array (concatenate)(w198, w199, w197, w196, w195, w194, w193, w192, w191, w190, w189, w188, w187, w186, w185, w184, w183, w182, w181, w180, w179) -> (w178:refnum<vi>[])
      n198 = control-ref of="BOB4FVBin_MonData"() -> (w177:refnum<vi>)
      n199 = control-ref of="BOB5GVSin_MonData"() -> (w176:refnum<vi>)
      n200 = control-ref of="BOB5GVPin_MonData"() -> (w175:refnum<vi>)
      n201 = control-ref of="BOB5TPin_MonData"() -> (w174:refnum<vi>)
      n202 = control-ref of="BOB5FCin_MonData"() -> (w173:refnum<vi>)
      n203 = control-ref of="BOB5MCPin_MonData"() -> (w172:refnum<vi>)
      n204 = control-ref of="BOB5FVAin_MonData"() -> (w171:refnum<vi>)
      n205 = control-ref of="BOB5FVBin_MonData"() -> (w170:refnum<vi>)
      n206 = control-ref of="PT1GVPin_MonData"() -> (w169:refnum<vi>)
      n207 = control-ref of="PT1TPin_MonData"() -> (w168:refnum<vi>)
      n208 = control-ref of="PT1FVAin_MonData"() -> (w167:refnum<vi>)
      n209 = control-ref of="PT1FVBin_MonData"() -> (w166:refnum<vi>)
      n210 = control-ref of="PT2GVPin_MonData"() -> (w165:refnum<vi>)
      n211 = control-ref of="PT2TPin_MonData"() -> (w164:refnum<vi>)
      n212 = control-ref of="PT2FVAin_MonData"() -> (w163:refnum<vi>)
      n213 = control-ref of="PT2FVBin_MonData"() -> (w162:refnum<vi>)
      n214 = Build Array (concatenate)(w178, w177, w176, w175, w174, w173, w172, w171, w170, w169, w168, w167, w166, w165, w164, w163, w162) -> (w161:refnum<vi>[])
      n215 = for "Subscribe to DIM MON Values in" {
        tunnel: w161 -> [w217] mode=indexing
        tunnel: w161 -> [w221] mode=indexing
        n216 = property class="Clust (strict)"(reference=w217) -> ("Label.Text"=w220:string)  [unwired: 1 in, 2 out]
        n217 = Match Pattern(string=w220, regular expression="Data") -> (before substring=w218:string)  [unwired: 1 in, 3 out]
        n218 = call "DimIndicators.dic_info_service.vi"("controlRef"=w221, "serviceName"=w218) -> ()  [unwired: 16 in, 2 out]
      }
    }
    frame #6 {
      # "DIM Mon Values Variables  (Boolean Out)"
      n219 = control-ref of="TSTGVSout_MonData"() -> (w265:refnum<vi>)
      n220 = control-ref of="TSTTPout_MonData"() -> (w264:refnum<vi>)
      n221 = control-ref of="TSTFVAout_MonData"() -> (w263:refnum<vi>)
      n222 = control-ref of="TSTFVBout_MonData"() -> (w262:refnum<vi>)
      n223 = control-ref of="BOB2TISout_MonData"() -> (w222:refnum<vi>)
      n224 = control-ref of="BOB1FCout_MonData"() -> (w278:refnum<vi>)
      n225 = control-ref of="BOB1FVAout_MonData"() -> (w277:refnum<vi>)
      n226 = control-ref of="BOB1FVBout_MonData"() -> (w276:refnum<vi>)
      n227 = control-ref of="BOB1GVPout_MonData"() -> (w275:refnum<vi>)
      n228 = control-ref of="BOB1GVSout_MonData"() -> (w274:refnum<vi>)
      n229 = control-ref of="BOB1BETAout_MonData"() -> (w273:refnum<vi>)
      n230 = control-ref of="BOB1TPout_MonData"() -> (w272:refnum<vi>)
      n231 = control-ref of="BOB2FCout_MonData"() -> (w271:refnum<vi>)
      n232 = control-ref of="BOB2FVAout_MonData"() -> (w270:refnum<vi>)
      n233 = control-ref of="BOB2FVBout_MonData"() -> (w269:refnum<vi>)
      n234 = control-ref of="BOB2GVPout_MonData"() -> (w268:refnum<vi>)
      n235 = control-ref of="BOB2GVSout_MonData"() -> (w267:refnum<vi>)
      n236 = control-ref of="BOB2TPout_MonData"() -> (w266:refnum<vi>)
      n237 = Build Array(w278, w277, w276, w275, w274, w273, w272, w271, w270, w269, w268, w267, w266, w265, w264, w263, w262, w222) -> (w260:refnum<vi>[])
      n238 = control-ref of="BOB3GVSout_MonData"() -> (w261:refnum<vi>)
      n239 = control-ref of="BOB3GVPout_MonData"() -> (w259:refnum<vi>)
      n240 = control-ref of="BOB3TPout_MonData"() -> (w258:refnum<vi>)
      n241 = control-ref of="BOB3FCout_MonData"() -> (w257:refnum<vi>)
      n242 = control-ref of="BOB3MCPout_MonData"() -> (w256:refnum<vi>)
      n243 = control-ref of="BOB3FVAout_MonData"() -> (w255:refnum<vi>)
      n244 = control-ref of="BOB3FVBout_MonData"() -> (w254:refnum<vi>)
      n245 = control-ref of="CBFVAout_MonData"() -> (w253:refnum<vi>)
      n246 = control-ref of="CBFVBout_MonData"() -> (w252:refnum<vi>)
      n247 = control-ref of="CBFVCout_MonData"() -> (w251:refnum<vi>)
      n248 = control-ref of="CB1TPout_MonData"() -> (w250:refnum<vi>)
      n249 = control-ref of="CB2TPout_MonData"() -> (w249:refnum<vi>)
      n250 = control-ref of="CB3TPout_MonData"() -> (w248:refnum<vi>)
      n251 = control-ref of="CB4TPout_MonData"() -> (w247:refnum<vi>)
      n252 = control-ref of="CB5GVSout_MonData"() -> (w246:refnum<vi>)
      n253 = control-ref of="BOB4GVSout_MonData"() -> (w245:refnum<vi>)
      n254 = control-ref of="BOB4GVPout_MonData"() -> (w244:refnum<vi>)
      n255 = control-ref of="BOB4TPout_MonData"() -> (w243:refnum<vi>)
      n256 = control-ref of="BOB4BETAout_MonData"() -> (w242:refnum<vi>)
      n257 = control-ref of="BOB4FVAout_MonData"() -> (w241:refnum<vi>)
      n258 = Build Array (concatenate)(w260, w261, w259, w258, w257, w256, w255, w254, w253, w252, w251, w250, w249, w248, w247, w246, w245, w244, w243, w242, w241) -> (w240:refnum<vi>[])
      n259 = control-ref of="BOB4FVBout_MonData"() -> (w239:refnum<vi>)
      n260 = control-ref of="BOB5GVSout_MonData"() -> (w238:refnum<vi>)
      n261 = control-ref of="BOB5GVPout_MonData"() -> (w237:refnum<vi>)
      n262 = control-ref of="BOB5TPout_MonData"() -> (w236:refnum<vi>)
      n263 = control-ref of="BOB5FCout_MonData"() -> (w235:refnum<vi>)
      n264 = control-ref of="BOB5MCPout_MonData"() -> (w234:refnum<vi>)
      n265 = control-ref of="BOB5FVAout_MonData"() -> (w233:refnum<vi>)
      n266 = control-ref of="BOB5FVBout_MonData"() -> (w232:refnum<vi>)
      n267 = control-ref of="PT1GVPout_MonData"() -> (w231:refnum<vi>)
      n268 = control-ref of="PT1TPout_MonData"() -> (w230:refnum<vi>)
      n269 = control-ref of="PT1FVAout_MonData"() -> (w229:refnum<vi>)
      n270 = control-ref of="PT1FVBout_MonData"() -> (w228:refnum<vi>)
      n271 = control-ref of="PT2GVPout_MonData"() -> (w227:refnum<vi>)
      n272 = control-ref of="PT2TPout_MonData"() -> (w226:refnum<vi>)
      n273 = control-ref of="PT2FVAout_MonData"() -> (w225:refnum<vi>)
      n274 = control-ref of="PT2FVBout_MonData"() -> (w224:refnum<vi>)
      n275 = Build Array (concatenate)(w240, w239, w238, w237, w236, w235, w234, w233, w232, w231, w230, w229, w228, w227, w226, w225, w224) -> (w223:refnum<vi>[])
      n276 = for "Subscribe to DIM MON Values Out" {
        tunnel: w223 -> [w279] mode=indexing
        tunnel: w223 -> [w283] mode=indexing
        n277 = property class="Clust (strict)"(reference=w279) -> ("Label.Text"=w282:string)  [unwired: 1 in, 2 out]
        n278 = Match Pattern(string=w282, regular expression="Data") -> (before substring=w280:string)  [unwired: 1 in, 3 out]
        n279 = call "DimIndicators.dic_info_service.vi"("controlRef"=w283, "serviceName"=w280) -> ()  [unwired: 16 in, 2 out]
      }
    }
    frame #7 {
      # "DIM Set Values Variables (Boolean)"
      n280 = control-ref of="BOB1lock_SetData"() -> (w292:refnum<vi>)
      n281 = control-ref of="BOB2lock_SetData"() -> (w291:refnum<vi>)
      n282 = control-ref of="BOB3lock_SetData"() -> (w290:refnum<vi>)
      n283 = control-ref of="BOB4lock_SetData"() -> (w289:refnum<vi>)
      n284 = control-ref of="BOB5lock_SetData"() -> (w288:refnum<vi>)
      n285 = control-ref of="TSTlock_SetData"() -> (w287:refnum<vi>)
      n286 = control-ref of="CBlock_SetData"() -> (w286:refnum<vi>)
      n287 = control-ref of="PTlock_SetData"() -> (w285:refnum<vi>)
      n288 = Build Array(w292, w291, w290, w289, w288, w287, w286, w285) -> (w284:refnum<vi>[])
      n289 = for "Subscribe to DIM Set Values" {
        tunnel: w284 -> [w293] mode=indexing
        tunnel: w284 -> [w297] mode=indexing
        n290 = property class="Clust (strict)"(reference=w293) -> ("Label.Text"=w296:string)  [unwired: 1 in, 2 out]
        n291 = Match Pattern(string=w296, regular expression="Data") -> (before substring=w294:string)  [unwired: 1 in, 3 out]
        n292 = call "DimIndicators.dic_info_service.vi"("controlRef"=w297, "serviceName"=w294) -> ()  [unwired: 16 in, 2 out]
      }
    }
    frame #8 {
      # "DIM Monitor Values Variables (Numeric)"
      n293 = control-ref of="BOB5PEN_MonData"() -> (w305:refnum<vi>)
      n294 = control-ref of="BOB1PEN_MonData"() -> (w311:refnum<vi>)
      n295 = control-ref of="BOB1PIR_MonData"() -> (w312:refnum<vi>)
      n296 = control-ref of="BOB2PEN_MonData"() -> (w313:refnum<vi>)
      n297 = control-ref of="BOB2PIR_MonData"() -> (w319:refnum<vi>)
      n298 = control-ref of="BOB3PEN_MonData"() -> (w318:refnum<vi>)
      n299 = control-ref of="BOB3PIR_MonData"() -> (w327:refnum<vi>)
      n300 = control-ref of="BOB3_MCP_MonData"() -> (w326:refnum<vi>)
      n301 = control-ref of="BOB3_Pho_MonData"() -> (w325:refnum<vi>)
      n302 = control-ref of="CB1PEN_MonData"() -> (w324:refnum<vi>)
      n303 = control-ref of="CB2PEN_MonData"() -> (w323:refnum<vi>)
      n304 = control-ref of="CB3PEN_MonData"() -> (w322:refnum<vi>)
      n305 = control-ref of="BOB4PEN_MonData"() -> (w321:refnum<vi>)
      n306 = control-ref of="BOB4PIR_MonData"() -> (w320:refnum<vi>)
      n307 = control-ref of="BOB5_MCP_MonData"() -> (w307:refnum<vi>)
      n308 = control-ref of="BOB5_Pho_MonData"() -> (w306:refnum<vi>)
      n309 = control-ref of="BOB5PIR_MonData"() -> (w317:refnum<vi>)
      n310 = control-ref of="PT1PEN_MonData"() -> (w316:refnum<vi>)
      n311 = control-ref of="PT1PIR_MonData"() -> (w315:refnum<vi>)
      n312 = control-ref of="BOB6_MCP_MonData"() -> (w314:refnum<vi>)
      n313 = control-ref of="BOB6_Pho_MonData"() -> (w310:refnum<vi>)
      n314 = control-ref of="PT2PEN_MonData"() -> (w309:refnum<vi>)
      n315 = control-ref of="PT2PIR_MonData"() -> (w308:refnum<vi>)
      n316 = control-ref of="FVAPIR_MonData"() -> (w303:refnum<vi>)
      n317 = control-ref of="FVBPIR_MonData"() -> (w302:refnum<vi>)
      n318 = control-ref of="LN2Level_MonData"() -> (w300:refnum<vi>)
      n319 = control-ref of="LHeLevel_MonData"() -> (w299:refnum<vi>)
      n320 = control-ref of="FVCPIR_MonData"() -> (w298:refnum<vi>)
      n321 = Build Array(w311, w312, w313, w319, w318, w327, w326, w325, w324, w323, w322, w321, w320, w307, w306, w305) -> (w304:refnum<vi>[])
      n322 = Build Array (concatenate)(w304, w317, w316, w315, w314, w310, w309, w308, w303, w302, w300, w299, w298) -> (w301:refnum<vi>[])
      n323 = for "Subscribe to DIM  Monitor Values (Numeric)" {
        tunnel: w301 -> [w328] mode=indexing
        tunnel: w301 -> [w332] mode=indexing
        n324 = property class="Clust (strict)"(reference=w328) -> ("Label.Text"=w331:string)  [unwired: 1 in, 2 out]
        n325 = Match Pattern(string=w331, regular expression="Data") -> (before substring=w329:string)  [unwired: 1 in, 3 out]
        n326 = call "DimIndicators.dic_info_service.vi"("controlRef"=w332, "serviceName"=w329) -> ()  [unwired: 16 in, 2 out]
      }
    }
    frame #9 {
      # "Reason For Locking a section indicator and DIM variable are created here"
      # "DIM Set Values Variables"
      n327 = control-ref of="BOB5_MCP_SetData"() -> (w338:refnum<vi>)
      n328 = control-ref of="BOB6_Pho_SetData"() -> (w337:refnum<vi>)
      n329 = control-ref of="BOB6_MCP_SetData"() -> (w336:refnum<vi>)
      n330 = control-ref of="BOB3_Pho_SetData"() -> (w341:refnum<vi>)
      n331 = control-ref of="BOB3_MCP_SetData"() -> (w340:refnum<vi>)
      n332 = control-ref of="BOB5_Pho_SetData"() -> (w339:refnum<vi>)
      n333 = control-ref of="ReasonForLocking_SetData"() -> (w333:refnum<vi>)
      n334 = Build Array(w341, w340, w339, w338, w337, w336) -> (w335:refnum<vi>[])
      n335 = for "Subscribe to DIM Set Values" {
        tunnel: w335 -> [w345] mode=indexing
        n336 = property class="Clust (strict)"(reference=w345) -> ("Label.Text"=w344:string)  [unwired: 1 in, 2 out]
        n337 = Match Pattern(string=w344, regular expression="Data") -> (before substring=w342:string)  [unwired: 1 in, 3 out]
        n338 = call "DimIndicators.dic_info_service.vi"("controlRef"=w345, "serviceName"=w342) -> ()  [unwired: 16 in, 2 out]
      }
      n339 = call "DimIndicators.dic_info_service.vi"("controlRef"=w333, "serviceName"="ReasonForLocking") -> ()  [unwired: 16 in, 2 out]
    }
    frame #10 {
      # "Sort Control Arrays"
      n340 = call "SortArraysVac.vi"("EnIndicators"=w347, "DIMControSet"=w353, "DIMControlMon out"=w354, "DIMControlMon in"=w355, "FPIndicator"=w361) -> ("Boolean (Strict) (sorted)"=w346:refnum<vi>[], "DIMControSet (sorted)"=w352:refnum<vi>[], "DIMControlMon out (sorted)"=w350:refnum<vi>[], "DIMControlMon in (sorted)"=w351:refnum<vi>[], "FPIndicator sorted"=w360:refnum<vi>[])  [unwired: 17 in, 1 out]
      n341 = call "SortArraysPLC.vi"("FPIndicator in"=w359, "DIMControlMon"=w358, "DIMControSet"=w349) -> ("FPIndicator out"=w357:refnum<vi>[], "DIMControlMon out"=w356:refnum<vi>[], "DIMControSet out"=w348:refnum<vi>[])  [unwired: 20 in, 2 out]
    }
    frame #11 {
      n342 = while "Wait For User Commands and Variable Changes" {
        tunnel: w367 -> [w380]
        tunnel: w368 -> [w379]
        tunnel: w370 -> [w373]
        tunnel: w369 -> [w377]
        tunnel: w366 -> [w376]
        tunnel: w365 -> [w375]
        tunnel: w364 -> [w374]
        tunnel: w363 -> [w372]
        tunnel: w362 -> [w371]
        stop <- w381 stop-if-true
        n343 = event "Act on User Selection or Variable Changes" shown="[11] \"ReasonForLocking_SetData\": Value Change" {
          selector: _ -> [_ _ _ _ _ _ _ _ _ _ _ _ _]
          dyn-events: _ -> [_ _ _ _ _ _ _ _ _ _ _ _ _]
          timeout: -1 -> [_ _ _ _ _ _ _ _ _ _ _ _ _]
          tunnel: [_ w382 _ _ _ _ _ _ _ _ _ _ TRUE ("stop")] -> w381
          tunnel: w380 -> [_ _ w398 w420 _ _ _ _ w564 _ _ _ w785]
          tunnel: w379 -> [_ _ w397 w419 _ _ _ _ _ w659 _ _ w786]
          tunnel: w377 -> [_ _ _ _ _ _ _ _ _ _ w755 _ w788]
          tunnel: w376 -> [_ _ w400 w425 w450 _ w484 _ _ _ _ _ w784]
          tunnel: w375 -> [_ _ w396 w423 w457 _ w486 _ w565 w661 _ _ _]
          tunnel: w374 -> [_ _ _ _ _ _ _ _ _ _ _ _ w787]
          tunnel: w373 -> [_ _ _ _ _ _ _ _ _ _ w754 _ _]
          tunnel: w372 -> [_ _ _ w428 _ _ _ _ _ _ _ _ w789]
          tunnel: w371 -> [_ _ _ _ _ _ _ _ w563 w658 _ _ _]
          event Timeout {
            # "Timeout"
            n344 = event-data() -> ()  [unwired: 1 in, 3 out]
          }
          event Menu Selection (User) {
            # "Deal With Menu Selections"
            n345 = event-data() -> ("ItemTag"=w383:string)  [unwired: 1 in]
            n346 = case "Selection?" shown="\"VacSymbols\"" w383 {
              tunnel: [_ _ _ _ TRUE ("stop")] -> w382
              frame "False", Default {
              }
              frame "Legend" {
                # "Open Legend"
                n347 = call "VacLegend.vi"("i ref in"=refnum<vi> refnum) -> ("i ref out"=→"i ref out":refnum<vi>)  [unwired: 10 in]
              }
              frame "VacSafety" {
                # "Open Vacuum Saftey Legend"
                n348 = call "VacSafety.vi"("i ref in"=refnum<vi> refnum) -> ("i ref out"=→"i ref out":refnum<vi>)  [unwired: 10 in]
              }
              frame "VacSymbols" {
                n349 = call "VacSymbols.vi"("i ref in"=refnum<vi> refnum) -> ("i ref out"=→"i ref out":refnum<vi>)  [unwired: 10 in]
              }
              frame "BUNAPP_FILE_EXIT" {
                # "Exit"
              }
            }
          }
          event "BOB1BETA", "BOB1FC", "BOB6FC", "BOB3FC", "BOB2FC", "BOB5FC", "BOB4BETA", "BOB1GVS", "TSTGVS", "BOB2GVS", "BOB3GVS", "BOB4GVS", "BOB5GVS", "BOB1GVP", "BOB2GVP", "BOB3GVP", "CB5GVS", "BOB4GVP", "BOB5GVP", "PT1GVP", "PT2GVP", "BOB1FVA", "BOB1FVB", "BOB2FVA", "BOB2FVB", "TSTFVA", "TSTFVB", "BOB3FVA", "BOB3FVB", "CBFVA", "CBFVC", "CBFVB", "BOB4FVA", "BOB4FVB", "BOB5FVA", "BOB5FVB", "PT1FVA", "PT1FVB", "PT2FVA", "PT2FVB", "BOB3TP", "TSTTP", "CB1TP", "BOB2TP", "BOB1TP", "BOB5TP", "PT2TP", "BOB4TP", "PT1TP", "BOB2TIS": Mouse Down {
            # "Find Indicator Index"
            # "Only the Prevacs, Gate Values and Turbo\npumps have enable relays"
            n350 = event-data() -> ("CtlRef"=w393:refnum<vi>)  [unwired: 1 in, 5 out]
            n351 = property class="Bool (strict)"(reference=w393) -> ("Label.Text"=w399:string)  [unwired: 1 in, 2 out]
            n352 = Search 1D Array(1D array=w396, element=w393) -> (index of element=w394:i32)  [unwired: 1 in]
            n353 = call "SectionLocked.vi"("Control Name"=w399, "DIMControSet (Locks)"=w400) -> ("Linked?"=w392:bool, "Unlocked?"=w395:bool)
            n354 = case "Section Unlocked?" shown="True" w395 {
              tunnel: w399 -> [_ w402]
              tunnel: string[] ["FVA", "FVB", "FVC", "GVP", "GVS", "TP"] -> [_ w404]
              tunnel: w398 -> [_ w407]
              tunnel: w397 -> [_ w408]
              tunnel: w394 -> [_ w406]
              tunnel: w392 -> [w401 _]
              frame False {
                # "Display Message to the User"
                n355 = call "Display Message to User"("Enable"=w401) -> ()  [unwired: 9 in, 2 out]
              }
              frame True {
                n356 = Array Size(array=w404) -> (size(s)=w403:i32)
                n357 = while "Determine if the indicator \nhas an enable relay" {
                  tunnel: w404 -> [w416] mode=indexing
                  tunnel: w402 -> [w415]
                  tunnel: [w412] -> w405
                  tunnel: w403 -> [w410]
                  i -> [w414]
                  stop <- w413 stop-if-true
                  n358 = Decrement(x=w410) -> (x-1=w409:i32)
                  n359 = Match Pattern(string=w415, regular expression=w416) -> (offset past match=w417:i32)  [unwired: 1 in, 3 out]
                  n360 = Not Equal?(x=w417, y=-1) -> (x != y?=w412:bool)
                  n361 = Equal?(x=w414, y=w409) -> (x = y?=w411:bool)
                  n362 = Or(x=w412, y=w411) -> (x .or. y?=w413:bool)
                }
                n363 = call "UpdateVacPLC.vi"("index of element"=w406, "DIMControlMon in (sorted)"=w408, "DIMControlMon out (sorted)"=w407, "Label.Text"=w402, "Enable?"=w405) -> ()  [unwired: 15 in]
              }
            }
          }
          event "BOB5MCP", "BOB3MCP", "BOB6MCP": Mouse Down {
            # "Find Indicator Index"
            n364 = event-data() -> ("CtlRef"=w422:refnum<vi>)  [unwired: 1 in, 7 out]
            n365 = property class="Bool (strict)"(reference=w422) -> ("Label.Text"=w426:string, "Value"=w429:bool)  [unwired: 1 in, 2 out]
            n366 = Search 1D Array(1D array=w423, element=w422) -> (index of element=w421:i32)  [unwired: 1 in]
            n367 = call "SectionLocked.vi"("Control Name"=w426, "DIMControSet (Locks)"=w425) -> ("Linked?"=w424:bool, "Unlocked?"=w427:bool)
            n368 = case "Section Unlocked?" shown="True" w427 {
              tunnel: w426 -> [_ w436]
              tunnel: w429 -> [_ w438]
              tunnel: w428 -> [_ w437]
              tunnel: w424 -> [w430 _]
              tunnel: w421 -> [_ w435]
              tunnel: w420 -> [_ w434]
              tunnel: w419 -> [_ w433]
              frame False {
                # "Section Locked"
                n369 = call "Display Message to User"("Enable"=w430) -> ()  [unwired: 9 in, 2 out]
              }
              frame True {
                n370 = call "CheckMCP.vi"("MCP Control Name"=w436, "MCP_DIM_SetData"=w437) -> ("No Link?"=w431:bool, "Safe?"=w432:bool)
                n371 = case "No Link?" shown="False" w431 {
                  tunnel: w438 -> [w444 _]
                  tunnel: w436 -> [w443 _]
                  tunnel: w435 -> [w442 _]
                  tunnel: w434 -> [w441 _]
                  tunnel: w433 -> [w440 _]
                  tunnel: w432 -> [w439 _]
                  frame False {
                    n372 = case "MCP Safe?" shown="True" w439 {
                      tunnel: w444 -> [_ _]
                      tunnel: w443 -> [_ w445]
                      tunnel: w442 -> [_ w448]
                      tunnel: w441 -> [_ w447]
                      tunnel: w440 -> [_ w446]
                      frame False {
                        # "MCP Not Safe"
                        n373 = call "Display Message to User"() -> ()  [unwired: 10 in, 2 out]
                      }
                      frame True {
                        # "Change MCP Position"
                        n374 = call "UpdateVacPLC.vi"("index of element"=w448, "DIMControlMon in (sorted)"=w446, "DIMControlMon out (sorted)"=w447, "Label.Text"=w445, "Enable?"=FALSE) -> ()  [unwired: 15 in]
                      }
                    }
                  }
                  frame True {
                    # "Display Message to the User"
                    n375 = call "Display Message to User"() -> ()  [unwired: 10 in, 2 out]
                  }
                }
              }
            }
          }
          event "BOB1lock", "BOB2lock", "CBlock", "PTlock", "BOB5lock", "BOB4lock", "BOB3lock", "TSTlock": Mouse Down; "BOB1lock", "BOB2lock", "TSTlock", "PTlock", "CBlock", "BOB4lock", "BOB5lock", "BOB3lock": Value Change {
            # "Find Set Index"
            n376 = event-data() -> ("CtlRef"=w458:refnum<vi>)  [unwired: 1 in]
            n377 = property class="Bool (strict)"(reference=w458) -> ("Label.Text"=w451:string)  [unwired: 1 in, 2 out]
            n378 = Search 1D Array(1D array=w457, element=w458) -> (index of element=w456:i32)  [unwired: 1 in]
            n379 = Index Array(array=w450, index=w456) -> (element=w455:refnum<vi>)
            n380 = property class="Clust (strict)"(reference=w455) -> ("Value"=w454:T8)  [unwired: 1 in, 2 out]
            n381 = Unbundle By Name(w454) -> ("no link"=w453:bool, "data"=w452:i16)
            n382 = case "No Link?" shown="False" w453 {
              tunnel: w452 -> [w464 _]
              tunnel: w451 -> [w462 _]
              frame False {
                # "Safety Overwrite Off"
                # "Update Vacuum PLC"
                n383 = Less Or Equal To 0?(x=w464) -> (x <= 0?=w463:bool)
                n384 = Boolean To (0,1)(Boolean=w463) -> (0, 1=w465:i16)
                n385 = call-poly "CoreLib.data 2 byte array.vi"("i16"=w465) -> ("byteArray out"=w460:T4)  [unwired: 18 in]
                n386 = Concatenate Strings("SetVacuum" ("string"), w462) -> (w467:string)
                n387 = call-poly "CoreLib.data 2 byte array.vi"("byteArray"=w460, "i16"=i16 0) -> ("byteArray out"=w461:T4)  [unwired: 17 in]
                n388 = Bundle By Name(cluster="call cluster in", "Object"="VacuumPLC", "Selector"=w467, "CallType"=enum16{"simple", "synchronous", "asynchronous"}."simple", "Data"=w461) -> (w470:T2)
                n389 = call "CoreLib.call process.vi"("call cluster in"=w470) -> ()  [unwired: 13 in, 2 out]
              }
              frame True {
                # "No Link"
                n390 = call "Display Message to User"() -> ()  [unwired: 10 in, 2 out]
              }
            }
          }
          event "Reason for locking": Value Change {
            # "Update Vacuum PLC"
            n391 = event-data() -> ("CtlRef"=w479:refnum<vi>)  [unwired: 1 in, 3 out]
            n392 = property class="Str"(reference=w479) -> ("Value"=w473:string)  [unwired: 1 in, 2 out]
            n393 = call "EmptyString.vi"() -> ("String"=w476:string)
            n394 = Concatenate Strings(w473, "\r\n") -> (w475:string)
            n395 = Replace Substring(4:w475, 5:w476) -> (1:w477:string)  [unwired: 2 in, 1 out]
            n396 = call-poly "CoreLib.data 2 byte array.vi"("string"=w477) -> ("byteArray out"=w472:T4)  [unwired: 18 in]
            n397 = Bundle By Name(cluster="call cluster in", "Object"="VacuumPLC", "Selector"="SetLockingReason", "CallType"=enum16{"simple", "synchronous", "asynchronous"}."simple", "Data"=w472) -> (w482:T2)
            n398 = call "CoreLib.call process.vi"("call cluster in"=w482) -> ()  [unwired: 13 in, 2 out]
          }
          event Value Change {
            n399 = event-data() -> ("CtlRef"=w485:refnum<vi>, "NewVal"=w487:T1)  [unwired: 1 in, 5 out]
            n400 = stacked-sequence "Check and update section locks" {
              tunnel: w487 -> [w490 _]
              tunnel: w486 -> [w489 _]
              tunnel: w485 -> [w488 _]
              tunnel: w484 -> [_ w512]
              frame #0 {
                n401 = for "Check if Indicator Exists for the Set Value?" {
                  tunnel: w490 -> [w499]
                  tunnel: w488 -> [w496]
                  tunnel: w489 -> [w491] mode=indexing
                  n402 = property class="Bool (strict)"(reference=w491) -> (reference out=w492:refnum<vi>, "Label.Text"=w494:string)  [unwired: 1 in, 1 out]
                  n403 = property class="Clust (strict)"(reference=w496) -> ("Label.Text"=w497:string)  [unwired: 1 in, 2 out]
                  n404 = Match Pattern(string=w497, regular expression="_SetData") -> (before substring=w493:string)  [unwired: 1 in, 3 out]
                  n405 = Equal?(x=w494, y=w493) -> (x = y?=w495:bool)
                  n406 = case "Indicator exists?" shown="True" w495 {
                    tunnel: w499 -> [w505 _]
                    tunnel: w492 -> [w504 _]
                    frame True {
                      # "Updating a Section Lock"
                      n407 = Unbundle By Name(w505) -> ("data"=w502:dbl, "no link"=w501:bool)
                      n408 = case "No Link?" shown="False" w501 {
                        tunnel: w502 -> [w507 _]
                        tunnel: [w509 FALSE] -> w503
                        tunnel: [cluster{u32, u32}[] [{1985280, 1985280}, {6618880, 6618880}, {11245188, 10125428}] ("Colors [4]") cluster{u32, u32}[] [{16448250, 16448250}, {16448250, 16448250}, {11245188, 10125428}] ("Colors [4]")] -> w500
                        frame False {
                          n409 = Equal?(x=w507, y=i16 1) -> (x = y?=w509:bool)
                        }
                        frame True {
                        }
                      }
                      n410 = property on="Property Node" class="Bool (strict)"(reference=w504, "Value"=w503, "Colors [4]"=w500) -> ()  [unwired: 1 in, 2 out]
                    }
                    frame False {
                    }
                  }
                }
              }
              frame #1 {
                # "Check if any of the sections are locked to determine if\nthe reasons for locking string should be displayed"
                n411 = for "Check if any of the sections are locked" {
                  tunnel: w512 -> [w519] mode=indexing
                  shift-right: [w518] -> w513
                  shift-left: FALSE -> [w517]
                  n412 = property class="Clust (strict)"(reference=w519) -> ("Value"=w516:T8)  [unwired: 1 in, 2 out]
                  n413 = Unbundle By Name(w516) -> ("data"=w515:i16)
                  n414 = case "Section Locked?" shown="1" w515 {
                    tunnel: w517 -> [w520 _]
                    tunnel: [w520 TRUE] -> w518
                    frame 0, Default {
                    }
                    frame 1 {
                      # "Section locked\ndisplay reasons\nfor locking"
                    }
                  }
                }
                n415 = property on="Reason for locking" class="Str"("Visible"=w513) -> ()  [unwired: 2 in, 2 out]
              }
            }
          }
          event Value Change {
            # "Get NickName"
            # "Updating a Monitor Value"
            n416 = event-data() -> ("CtlRef"=w525:refnum<vi>, "NewVal"=w526:T1)  [unwired: 1 in, 5 out]
            n417 = property class="Clust (strict)"(reference=w525) -> ("Label.Text"=w523:string)  [unwired: 1 in, 2 out]
            n418 = Match Pattern(string=w523, regular expression="_MonData") -> (before substring=w522:string)  [unwired: 1 in, 3 out]
            n419 = case "Indicator exists?" shown="\"N4VAC\"" w522 {
              tunnel: w526 -> [w537 w555 _]
              frame "CB5SAFE" {
                n420 = Unbundle By Name(w537) -> ("data"=w532:dbl, "no link"=w528:bool, "quality"=w536:i32)
                n421 = Equal?(x=i16 -1, y=w532) -> (x = y?=w530:bool)
                n422 = Or(x=w530, y=w528) -> (x .or. y?=w529:bool)
                n423 = case shown="False" w528 {
                  tunnel: w536 -> [_ _]
                  tunnel: [w543 UtilityLib.valueStatus."no info available" ("valueStatus")] -> w535
                  tunnel: w532 -> [w541 _]
                  tunnel: [w542 _] -> w534
                  frame False {
                    n424 = call "CoreLib.quality 2 status.vi"("quality"=0) -> ("valueStatus"=w543:T7)  [unwired: 18 in]
                    n425 = Not Equal To 0?(x=w541) -> (x != 0?=w542:bool)
                  }
                  frame True {
                  }
                }
                n426 = case shown="False" w529 {
                  tunnel: [cluster{u32, u32}[] [{16711680, 16711680}, {6618880, 6618880}, {11245188, 10125428}] ("Colors [4]") cluster{u32, u32}[] [{16448250, 16448250}, {16448250, 16448250}, {11245188, 10125428}] ("Colors [4]")] -> w533
                  frame False {
                  }
                  frame True {
                  }
                }
                n427 = control-ref of="CB5SAFE"() -> (w527:refnum<vi>)
                n428 = property on="Property Node" class="Bool (strict)"(reference=w527, "Val(Sgnl)"=w534, "Colors [4]"=w533) -> ()  [unwired: 1 in, 2 out]
                n429 = call "TextColor(bool).vi"("valueStatus"=w535, "Ref"=w527) -> ()  [unwired: 10 in]
              }
              frame "N4VAC" {
                n430 = Unbundle By Name(w555) -> ("data"=w550:dbl, "no link"=w546:bool, "quality"=w554:i32)
                n431 = Equal?(x=i16 -1, y=w550) -> (x = y?=w548:bool)
                n432 = Or(x=w548, y=w546) -> (x .or. y?=w547:bool)
                n433 = case shown="False" w546 {
                  tunnel: w554 -> [_ _]
                  tunnel: [w561 UtilityLib.valueStatus."no info available" ("valueStatus")] -> w553
                  tunnel: w550 -> [w559 _]
                  tunnel: [w560 _] -> w552
                  frame False {
                    n434 = call "CoreLib.quality 2 status.vi"("quality"=0) -> ("valueStatus"=w561:T7)  [unwired: 18 in]
                    n435 = Not Equal To 0?(x=w559) -> (x != 0?=w560:bool)
                  }
                  frame True {
                  }
                }
                n436 = case shown="False" w547 {
                  tunnel: [cluster{u32, u32}[] [{16711680, 16711680}, {6618880, 6618880}, {11245188, 10125428}] ("Colors [4]") cluster{u32, u32}[] [{16448250, 16448250}, {16448250, 16448250}, {11245188, 10125428}] ("Colors [4]")] -> w551
                  frame False {
                  }
                  frame True {
                  }
                }
                n437 = control-ref of="N4VAC"() -> (w545:refnum<vi>)
                n438 = property on="Property Node" class="Bool (strict)"(reference=w545, "Val(Sgnl)"=w552, "Colors [4]"=w551) -> ()  [unwired: 1 in, 2 out]
                n439 = call "TextColor(bool).vi"("valueStatus"=w553, "Ref"=w545) -> ()  [unwired: 10 in]
              }
              frame Default {
              }
            }
          }
          event Value Change {
            n440 = event-data() -> ("CtlRef"=w566:refnum<vi>, "NewVal"=w567:T1)  [unwired: 1 in, 5 out]
            n441 = for "Check if Indicator Exists for the Monitor Value?" {
              tunnel: w567 -> [w583]
              tunnel: w566 -> [w580]
              tunnel: w565 -> [w577] mode=indexing
              tunnel: w564 -> [w576]
              tunnel: w563 -> [w573]
              i -> [w571]
              # "Updating a Monitor Value"
              n442 = property class="Bool (strict)"(reference=w577) -> (reference out=w568:refnum<vi>, "Label.Text"=w570:string)  [unwired: 1 in, 1 out]
              n443 = property class="Clust (strict)"(reference=w580) -> ("Label.Text"=w581:string)  [unwired: 1 in, 2 out]
              n444 = Index Array(array=w573, index=w571) -> (element=w572:refnum<vi>)
              n445 = Index Array(array=w576, index=w571) -> (element=w575:refnum<vi>)
              n446 = property class="Clust (strict)"(reference=w575) -> ("Value"=w574:T8)  [unwired: 1 in, 2 out]
              n447 = Match Pattern(string=w581, regular expression="in_MonData") -> (before substring=w578:string)  [unwired: 1 in, 3 out]
              n448 = Equal?(x=w570, y=w578) -> (x = y?=w579:bool)
              n449 = case "Indicator exists?" shown="True" w579 {
                tunnel: w583 -> [w605 _]
                tunnel: w568 -> [w603 _]
                tunnel: w574 -> [w602 _]
                tunnel: w572 -> [w590 _]
                tunnel: w570 -> [w585 _]
                tunnel: string[] ["FC", "MCP", "BETA", "TIS"] -> [w586 _]
                frame True {
                  n450 = Unbundle By Name(w602) -> ("data"=w594:i16, "no link"=w599:bool, "quality"=w598:i32)
                  n451 = Unbundle By Name(w605) -> ("data"=w595:dbl, "no link"=w600:bool, "quality"=w591:i32)
                  n452 = while "Is a Detector?" {
                    tunnel: w586 -> [w613] mode=indexing
                    tunnel: w585 -> [w614]
                    tunnel: [w606] -> w584
                    i -> [w612]
                    stop <- w608 stop-if-true
                    n453 = Match Pattern(string=w614, regular expression=w613) -> (offset past match=w610:i32)  [unwired: 1 in, 3 out]
                    n454 = Equal?(x=w612, y=3) -> (x = y?=w607:bool)
                    n455 = Not Equal?(x=-1, y=w610) -> (x != y?=w606:bool)
                    n456 = Or(x=w606, y=w607) -> (x .or. y?=w608:bool)
                  }
                  n457 = Multiply(x=i16 2, y=w594) -> (x*y=w593:i16)
                  n458 = Or(x=w599, y=w600) -> (x .or. y?=w601:bool)
                  n459 = Add(x=w593, y=w595) -> (x+y=w596:dbl)
                  n460 = case "No Link to DIM?" shown="False" w601 {
                    tunnel: [w616 UtilityLib.valueStatus."no info available" ("valueStatus")] -> w604
                    tunnel: [w622 cluster{u32, u32}[] [{16448250, 16448250}, {16448250, 16448250}, {11245188, 10125428}] ("Colors [4]")] -> w597
                    tunnel: w598 -> [w618 _]
                    tunnel: w596 -> [w621 _]
                    tunnel: [w620 w655] -> w592
                    tunnel: [w619 w655] -> w588
                    tunnel: w591 -> [w617 _]
                    tunnel: w584 -> [w615 _]
                    frame False {
                      n461 = case "Act on Monitors?" shown="1" w621 {
                        tunnel: [cluster{u32, u32}[] [{16776960, 16776960}, {16776960, 16776960}, {11245188, 10125428}] ("Colors [4]") w634 w638 cluster{u32, u32}[] [{16711680, 16711680}, {16711680, 16711680}, {11245188, 10125428}] ("Colors [4]") cluster{u32, u32}[] [{16448250, 16448250}, {16448250, 16448250}, {11245188, 10125428}] ("Colors [4]")] -> w622
                        tunnel: [FALSE TRUE FALSE FALSE w653] -> w620
                        tunnel: [TRUE w629 w639 TRUE w653] -> w619
                        tunnel: w618 -> [_ w631 _ _ _]
                        tunnel: w617 -> [w624 _ w640 w647 w651]
                        tunnel: [w625 w632 w641 w648 w652] -> w616
                        tunnel: w615 -> [_ w628 w637 _ _]
                        frame 0 {
                          # "In - False  Out - False"
                          n462 = call "CoreLib.quality 2 status.vi"("quality"=w624) -> ("valueStatus"=w625:T7)  [unwired: 18 in]
                        }
                        frame 1 {
                          # "In - True  Out - False"
                          n463 = case "Is a Detector?" shown="False" w628 {
                            tunnel: [cluster{u32, u32}[] [{6618880, 6618880}, {1985280, 1985280}, {11245188, 10125428}] ("Colors [4]") cluster{u32, u32}[] [{1985280, 1985280}, {6618880, 6618880}, {11245188, 10125428}] ("Colors [4]")] -> w634
                            frame False {
                            }
                            frame True {
                            }
                          }
                          n464 = Equal?(x=w631, y=3) -> (x = y?=w629:bool)
                          n465 = call "CoreLib.quality 2 status.vi"("quality"=w631) -> ("valueStatus"=w632:T7)  [unwired: 18 in]
                        }
                        frame 2 {
                          # "In - False  Out - True"
                          n466 = case "Is a Detector?" shown="True" w637 {
                            tunnel: [cluster{u32, u32}[] [{6618880, 6618880}, {1985280, 1985280}, {11245188, 10125428}] ("Colors [4]") cluster{u32, u32}[] [{1985280, 1985280}, {6618880, 6618880}, {11245188, 10125428}] ("Colors [4]")] -> w638
                            frame False {
                            }
                            frame True {
                            }
                          }
                          n467 = call "CoreLib.quality 2 status.vi"("quality"=w640) -> ("valueStatus"=w641:T7)  [unwired: 18 in]
                          n468 = Equal?(x=w640, y=3) -> (x = y?=w639:bool)
                        }
                        frame 3 {
                          # "In - True  Out - True"
                          n469 = call "CoreLib.quality 2 status.vi"("quality"=w647) -> ("valueStatus"=w648:T7)  [unwired: 18 in]
                        }
                        frame -2, -1, Default {
                          w653 = FALSE
                          # "No Link to DIM"
                          n470 = call "CoreLib.quality 2 status.vi"("quality"=w651) -> ("valueStatus"=w652:T7)  [unwired: 18 in]
                        }
                      }
                    }
                    frame True {
                      w655 = FALSE
                      # "No Link to DIM"
                    }
                  }
                  n471 = Not(x=w588) -> (.not. x?=w589:bool)
                  n472 = property on="Property Node" class="Bool (strict)"(reference=w603, "Colors [4]"=w597, "Val(Sgnl)"=w592) -> ()  [unwired: 1 in, 2 out]
                  n473 = property on="Property Node" class="Bool (strict)"(reference=w590, "Value"=w589) -> ()  [unwired: 1 in, 2 out]
                  n474 = call "TextColor(bool).vi"("valueStatus"=w604, "Ref"=w603) -> ()  [unwired: 10 in]
                }
                frame False {
                }
              }
            }
          }
          event Value Change {
            n475 = event-data() -> ("CtlRef"=w660:refnum<vi>, "NewVal"=w662:T1)  [unwired: 1 in, 5 out]
            n476 = for "Check if Indicator Exists for the Monitor Value?" {
              tunnel: w662 -> [w678]
              tunnel: w660 -> [w675]
              tunnel: w661 -> [w671] mode=indexing
              tunnel: w659 -> [w670]
              tunnel: w658 -> [w665]
              i -> [w667]
              # "Updating a Monitor Value"
              n477 = property class="Bool (strict)"(reference=w671) -> (reference out=w672:refnum<vi>, "Label.Text"=w664:string)  [unwired: 1 in, 1 out]
              n478 = property class="Clust (strict)"(reference=w675) -> ("Label.Text"=w676:string)  [unwired: 1 in, 2 out]
              n479 = Index Array(array=w670, index=w667) -> (element=w669:refnum<vi>)
              n480 = Index Array(array=w665, index=w667) -> (element=w666:refnum<vi>)
              n481 = property class="Clust (strict)"(reference=w669) -> ("Value"=w668:T8)  [unwired: 1 in, 2 out]
              n482 = Match Pattern(string=w676, regular expression="out_MonData") -> (before substring=w673:string)  [unwired: 1 in, 3 out]
              n483 = Equal?(x=w664, y=w673) -> (x = y?=w674:bool)
              n484 = case "Indicator exists?" shown="True" w674 {
                tunnel: w678 -> [w688 _]
                tunnel: w672 -> [w690 _]
                tunnel: w668 -> [w689 _]
                tunnel: w666 -> [w682 _]
                tunnel: w664 -> [w681 _]
                tunnel: string[] ["FC", "MCP", "BETA", "TIS"] -> [w680 _]
                frame True {
                  n485 = Unbundle By Name(w689) -> ("data"=w687:i16, "no link"=w694:bool, "quality"=w695:i32)
                  n486 = Unbundle By Name(w688) -> ("data"=w686:dbl, "no link"=w693:bool, "quality"=w700:i32)
                  n487 = while "Is a Detector?" {
                    tunnel: w680 -> [w708] mode=indexing
                    tunnel: w681 -> [w709]
                    tunnel: [w701] -> w679
                    i -> [w707]
                    stop <- w703 stop-if-true
                    n488 = Match Pattern(string=w709, regular expression=w708) -> (offset past match=w705:i32)  [unwired: 1 in, 3 out]
                    n489 = Equal?(x=w707, y=3) -> (x = y?=w702:bool)
                    n490 = Not Equal?(x=-1, y=w705) -> (x != y?=w701:bool)
                    n491 = Or(x=w701, y=w702) -> (x .or. y?=w703:bool)
                  }
                  n492 = Multiply(x=i16 2, y=w686) -> (x*y=w685:dbl)
                  n493 = Or(x=w694, y=w693) -> (x .or. y?=w692:bool)
                  n494 = Add(x=w687, y=w685) -> (x+y=w697:dbl)
                  n495 = case "No Link to DIM?" shown="False" w692 {
                    tunnel: [w711 UtilityLib.valueStatus."no info available" ("valueStatus")] -> w691
                    tunnel: [w717 cluster{u32, u32}[] [{16448250, 16448250}, {16448250, 16448250}, {11245188, 10125428}] ("Colors [4]")] -> w696
                    tunnel: w695 -> [w713 _]
                    tunnel: w697 -> [w716 _]
                    tunnel: [w715 w750] -> w699
                    tunnel: [w714 w750] -> w683
                    tunnel: w700 -> [w712 _]
                    tunnel: w679 -> [w710 _]
                    frame False {
                      n496 = case "Act on Monitors?" shown="-2, -1, Default" w716 {
                        tunnel: [cluster{u32, u32}[] [{16776960, 16776960}, {16776960, 16776960}, {11245188, 10125428}] ("Colors [4]") w724 w733 cluster{u32, u32}[] [{16711680, 16711680}, {16711680, 16711680}, {11245188, 10125428}] ("Colors [4]") cluster{u32, u32}[] [{16448250, 16448250}, {16448250, 16448250}, {11245188, 10125428}] ("Colors [4]")] -> w717
                        tunnel: [FALSE TRUE FALSE FALSE w748] -> w715
                        tunnel: [TRUE w727 w735 TRUE w748] -> w714
                        tunnel: w713 -> [_ _ w734 _ _]
                        tunnel: w712 -> [w719 w725 _ w742 w746]
                        tunnel: [w720 w728 w736 w743 w747] -> w711
                        tunnel: w710 -> [_ w723 w732 _ _]
                        frame 0 {
                          # "In - False  Out - False"
                          n497 = call "CoreLib.quality 2 status.vi"("quality"=w719) -> ("valueStatus"=w720:T7)  [unwired: 18 in]
                        }
                        frame 1 {
                          # "In - True  Out - False"
                          n498 = case "Is a Detector?" shown="False" w723 {
                            tunnel: [cluster{u32, u32}[] [{6618880, 6618880}, {1985280, 1985280}, {11245188, 10125428}] ("Colors [4]") cluster{u32, u32}[] [{1985280, 1985280}, {6618880, 6618880}, {11245188, 10125428}] ("Colors [4]")] -> w724
                            frame False {
                            }
                            frame True {
                            }
                          }
                          n499 = Equal?(x=w725, y=3) -> (x = y?=w727:bool)
                          n500 = call "CoreLib.quality 2 status.vi"("quality"=w725) -> ("valueStatus"=w728:T7)  [unwired: 18 in]
                        }
                        frame 2 {
                          # "In - False  Out - True"
                          n501 = case "Is a Detector?" shown="False" w732 {
                            tunnel: [cluster{u32, u32}[] [{6618880, 6618880}, {1985280, 1985280}, {11245188, 10125428}] ("Colors [4]") cluster{u32, u32}[] [{1985280, 1985280}, {6618880, 6618880}, {11245188, 10125428}] ("Colors [4]")] -> w733
                            frame False {
                            }
                            frame True {
                            }
                          }
                          n502 = call "CoreLib.quality 2 status.vi"("quality"=w734) -> ("valueStatus"=w736:T7)  [unwired: 18 in]
                          n503 = Equal?(x=w734, y=3) -> (x = y?=w735:bool)
                        }
                        frame 3 {
                          # "In - True  Out - True"
                          n504 = call "CoreLib.quality 2 status.vi"("quality"=w742) -> ("valueStatus"=w743:T7)  [unwired: 18 in]
                        }
                        frame -2, -1, Default {
                          w748 = FALSE
                          # "No Link to DIM"
                          n505 = call "CoreLib.quality 2 status.vi"("quality"=w746) -> ("valueStatus"=w747:T7)  [unwired: 18 in]
                        }
                      }
                    }
                    frame True {
                      w750 = FALSE
                      # "No Link to DIM"
                    }
                  }
                  n506 = Not(x=w683) -> (.not. x?=w684:bool)
                  n507 = property on="Property Node" class="Bool (strict)"(reference=w690, "Colors [4]"=w696, "Val(Sgnl)"=w699) -> ()  [unwired: 1 in, 2 out]
                  n508 = property on="Property Node" class="Bool (strict)"(reference=w682, "Value"=w684) -> ()  [unwired: 1 in, 2 out]
                  n509 = call "TextColor(bool).vi"("valueStatus"=w691, "Ref"=w690) -> ()  [unwired: 10 in]
                }
                frame False {
                }
              }
            }
          }
          event Value Change {
            # "Find Monitor Index"
            # "Updating a Numeric Monitor Value"
            n510 = event-data() -> ("CtlRef"=w756:refnum<vi>, "NewVal"=w757:T1)  [unwired: 1 in]
            n511 = Search 1D Array(1D array=w755, element=w756) -> (index of element=w759:i32)  [unwired: 1 in]
            n512 = Index Array(array=w754, index=w759) -> (element=w753:refnum<vi>)
            n513 = Not A Number/Path/Refnum?(number/path/refnum=w753) -> (NaN/Path/Refnum?=w758:bool)
            n514 = case "Indicator exists?" shown="False" w758 {
              tunnel: w757 -> [_ w766]
              tunnel: w753 -> [_ w760]
              frame True {
              }
              frame False {
                n515 = Unbundle By Name(w766) -> ("data"=w762:dbl, "no link"=w763:bool, "quality"=w765:i32)
                n516 = case "No Link?" shown="False" w763 {
                  tunnel: w765 -> [w769 _]
                  tunnel: [w768 UtilityLib.valueStatus."no info available" ("valueStatus")] -> w764
                  tunnel: w762 -> [w767 _]
                  tunnel: [w767 inf] -> w761
                  frame False {
                    n517 = call "CoreLib.quality 2 status.vi"("quality"=w769) -> ("valueStatus"=w768:T7)  [unwired: 18 in]
                  }
                  frame True {
                  }
                }
                n518 = property class="DigNum (strict)"(reference=w760, "Value"=w761) -> ()  [unwired: 1 in, 2 out]
                n519 = call "TextColor.vi"("valueStatus"=w764, "reference"=w760) -> ()  [unwired: 10 in]
              }
            }
          }
          event Value Change {
            # "Update Reason For Locking Indicator"
            n520 = event-data() -> ("NewVal"=w772:T5)  [unwired: 1 in]
            n521 = Unbundle By Name(w772) -> ("data"=w776:string, "no link"=w775:bool, "quality"=w774:i32)
            n522 = case "No Link?" shown="False" w775 {
              tunnel: w774 -> [w781 _]
              tunnel: [w780 UtilityLib.valueStatus."no info available" ("valueStatus")] -> w778
              tunnel: w776 -> [w779 _]
              tunnel: [w779 w782] -> w777
              frame False {
                n523 = call "CoreLib.quality 2 status.vi"("quality"=w781) -> ("valueStatus"=w780:T7)  [unwired: 18 in]
              }
              frame True {
                n524 = call "EmptyString.vi"() -> ("String"=w782:string)
              }
            }
            n525 = control-ref of="Reason for locking"() -> (w773:refnum<vi>)
            n526 = property class="Str"(reference=w773, "Value"=w777) -> ()  [unwired: 1 in, 2 out]
            n527 = call "UtilityLib.set color of GUI object.vi"("GUI object Ref"=w773, "valueStatus"=w778) -> ()  [unwired: 17 in, 1 out]
          }
          event Panel Close? {
            n528 = event-data() -> ()  [unwired: 1 in, 4 out]
            n529 = stacked-sequence {
              tunnel: w789 -> [w797 _]
              tunnel: w788 -> [w796 _]
              tunnel: w787 -> [w791 _]
              tunnel: w786 -> [w795 _]
              tunnel: w785 -> [w794 _]
              tunnel: w784 -> [w793 _]
              frame #0 {
                # "Release DIM Services"
                n530 = for "For Each Service" {
                  tunnel: w795 -> [w799] mode=indexing
                  n531 = Not A Number/Path/Refnum?(number/path/refnum=w799) -> (NaN/Path/Refnum?=w798:bool)
                  n532 = case "Not a Reference?" shown="False" w798 {
                    tunnel: w799 -> [w800 _]
                    frame False {
                      n533 = call "DimIndicators.dic_release_service.vi"("controlRef"=w800) -> ()  [unwired: 18 in, 1 out]
                    }
                    frame True {
                    }
                  }
                }
                n534 = for "For Each Service" {
                  tunnel: w793 -> [w805] mode=indexing
                  n535 = Not A Number/Path/Refnum?(number/path/refnum=w805) -> (NaN/Path/Refnum?=w804:bool)
                  n536 = case "Not a Reference?" shown="False" w804 {
                    tunnel: w805 -> [w806 _]
                    frame False {
                      n537 = call "DimIndicators.dic_release_service.vi"("controlRef"=w806) -> ()  [unwired: 18 in, 1 out]
                    }
                    frame True {
                    }
                  }
                }
                n538 = for "For Each Service" {
                  tunnel: w796 -> [w802] mode=indexing
                  n539 = Not A Number/Path/Refnum?(number/path/refnum=w802) -> (NaN/Path/Refnum?=w801:bool)
                  n540 = case "Not a Reference?" shown="False" w801 {
                    tunnel: w802 -> [w803 _]
                    frame False {
                      n541 = call "DimIndicators.dic_release_service.vi"("controlRef"=w803) -> ()  [unwired: 18 in, 1 out]
                    }
                    frame True {
                    }
                  }
                }
                n542 = control-ref of="ReasonForLocking_SetData"() -> (w792:refnum<vi>)
                n543 = for "For Each Service" {
                  tunnel: w797 -> [w814] mode=indexing
                  n544 = Not A Number/Path/Refnum?(number/path/refnum=w814) -> (NaN/Path/Refnum?=w813:bool)
                  n545 = case "Not a Reference?" shown="False" w813 {
                    tunnel: w814 -> [w815 _]
                    frame False {
                      n546 = call "DimIndicators.dic_release_service.vi"("controlRef"=w815) -> ()  [unwired: 18 in, 1 out]
                    }
                    frame True {
                    }
                  }
                }
                n547 = for "For Each Service" {
                  tunnel: w791 -> [w811] mode=indexing
                  n548 = Not A Number/Path/Refnum?(number/path/refnum=w811) -> (NaN/Path/Refnum?=w810:bool)
                  n549 = case "Not a Reference?" shown="False" w810 {
                    tunnel: w811 -> [w812 _]
                    frame False {
                      n550 = call "DimIndicators.dic_release_service.vi"("controlRef"=w812) -> ()  [unwired: 18 in, 1 out]
                    }
                    frame True {
                    }
                  }
                }
                n551 = for "For Each Service" {
                  tunnel: w794 -> [w808] mode=indexing
                  n552 = Not A Number/Path/Refnum?(number/path/refnum=w808) -> (NaN/Path/Refnum?=w807:bool)
                  n553 = case "Not a Reference?" shown="False" w807 {
                    tunnel: w808 -> [w809 _]
                    frame False {
                      n554 = call "DimIndicators.dic_release_service.vi"("controlRef"=w809) -> ()  [unwired: 18 in, 1 out]
                    }
                    frame True {
                    }
                  }
                }
                n555 = call "DimIndicators.dic_release_service.vi"("controlRef"=w792) -> ()  [unwired: 18 in, 1 out]
              }
              frame #1 {
                # "Close Front Panel"
                n556 = Current VI's Path() -> (path=w819:path)
                n557 = Open VI Reference(vi path=w819) -> (vi reference=w817:refnum<vi>, error out=w816:errorcluster)  [unwired: 5 in]
                n558 = property class="VI"(reference=w817, error in=w816, "Front Panel Window:Open"=FALSE) -> ()  [unwired: 2 out]
              }
            }
            n559 = event-data() -> ()  [unwired: 2 in, 1 out]
          }
        }
      }
    }
    frame #12 {
      n560 = stacked-sequence "Release DIM Variables" {
        tunnel: w824 -> [w830 _ _]
        tunnel: w825 -> [w831 _ _]
        tunnel: w823 -> [w829 _ _]
        tunnel: w822 -> [w828 _ _]
        tunnel: w821 -> [w832 _ _]
        tunnel: w820 -> [w826 _ _]
        frame #0 {
          # "Release DIM Services"
          n561 = for "For Each Service" {
            tunnel: w830 -> [w834] mode=indexing
            n562 = Not A Number/Path/Refnum?(number/path/refnum=w834) -> (NaN/Path/Refnum?=w833:bool)
            n563 = case "Not a Reference?" shown="False" w833 {
              tunnel: w834 -> [w835 _]
              frame False {
                n564 = call "DimIndicators.dic_release_service.vi"("controlRef"=w835) -> ()  [unwired: 18 in, 1 out]
              }
              frame True {
              }
            }
          }
          n565 = for "For Each Service" {
            tunnel: w828 -> [w840] mode=indexing
            n566 = Not A Number/Path/Refnum?(number/path/refnum=w840) -> (NaN/Path/Refnum?=w839:bool)
            n567 = case "Not a Reference?" shown="False" w839 {
              tunnel: w840 -> [w841 _]
              frame False {
                n568 = call "DimIndicators.dic_release_service.vi"("controlRef"=w841) -> ()  [unwired: 18 in, 1 out]
              }
              frame True {
              }
            }
          }
          n569 = for "For Each Service" {
            tunnel: w831 -> [w837] mode=indexing
            n570 = Not A Number/Path/Refnum?(number/path/refnum=w837) -> (NaN/Path/Refnum?=w836:bool)
            n571 = case "Not a Reference?" shown="False" w836 {
              tunnel: w837 -> [w838 _]
              frame False {
                n572 = call "DimIndicators.dic_release_service.vi"("controlRef"=w838) -> ()  [unwired: 18 in, 1 out]
              }
              frame True {
              }
            }
          }
          n573 = control-ref of="ReasonForLocking_SetData"() -> (w827:refnum<vi>)
          n574 = call "DimIndicators.dic_release_service.vi"("controlRef"=w827) -> ()  [unwired: 18 in, 1 out]
          n575 = for "For Each Service" {
            tunnel: w832 -> [w849] mode=indexing
            n576 = Not A Number/Path/Refnum?(number/path/refnum=w849) -> (NaN/Path/Refnum?=w848:bool)
            n577 = case "Not a Reference?" shown="False" w848 {
              tunnel: w849 -> [w850 _]
              frame False {
                n578 = call "DimIndicators.dic_release_service.vi"("controlRef"=w850) -> ()  [unwired: 18 in, 1 out]
              }
              frame True {
              }
            }
          }
          n579 = for "For Each Service" {
            tunnel: w826 -> [w846] mode=indexing
            n580 = Not A Number/Path/Refnum?(number/path/refnum=w846) -> (NaN/Path/Refnum?=w845:bool)
            n581 = case "Not a Reference?" shown="False" w845 {
              tunnel: w846 -> [w847 _]
              frame False {
                n582 = call "DimIndicators.dic_release_service.vi"("controlRef"=w847) -> ()  [unwired: 18 in, 1 out]
              }
              frame True {
              }
            }
          }
          n583 = for "For Each Service" {
            tunnel: w829 -> [w843] mode=indexing
            n584 = Not A Number/Path/Refnum?(number/path/refnum=w843) -> (NaN/Path/Refnum?=w842:bool)
            n585 = case "Not a Reference?" shown="False" w842 {
              tunnel: w843 -> [w844 _]
              frame False {
                n586 = call "DimIndicators.dic_release_service.vi"("controlRef"=w844) -> ()  [unwired: 18 in, 1 out]
              }
              frame True {
              }
            }
          }
        }
        frame #1 {
          # "Close Front Panel"
          n587 = Current VI's Path() -> (path=w854:path)
          n588 = Open VI Reference(vi path=w854) -> (vi reference=w852:refnum<vi>, error out=w851:errorcluster)  [unwired: 5 in]
          n589 = property class="VI"(reference=w852, error in=w851, "Front Panel Window:Open"=FALSE) -> ()  [unwired: 2 out]
        }
        frame #2 {
          # "Stop Panel"
          n590 = Stop(stop? (T)=TRUE) -> ()
        }
      }
    }
  }
  n591 = call "LVDimInterface.dim_operate.vi"("DNSNode"="lebit-balcony") -> ()  [unwired: 19 in]
